vi "I(V)_K2636B_PK.vi"() -> ()   [LabVIEW 2016]
uses:
  <instrlib>/Keithley 2600 Series/Public/Configure/Source/Configure Source (Limit).vi
  <instrlib>/Keithley 2600 Series/Public/Configure/Source/Configure Source (Range).vi
  <instrlib>/Keithley 2600 Series/Public/Data/Read Measurement (Current and Voltage).vi
  <instrlib>/Keithley 2600 Series/Keithley 2600 Series.lvlib
panel:
  in  "4-point sense":bool
  out "Resistance (ohm)":dbl=129228.0822461563 format="%#_13g"
  out "R vs V":cluster{dbl, "Field Reading":dbl}[](graph)=[{9.24826e-05, "Field Reading"=321246.1833983473}, {0.00208223, "Field Reading"=133422.3999282341}, {0.00408287, "Field Reading"=132230.99543994194}, {0.00608664, "Field Reading"=131799.94326658855}, {0.00808966, "Field Reading"=131627.15245472992}, {0.0100896, "Field Reading"=131526.7352701163}, {0.0120913, "Field Reading"=131453.46460596466}, {0.0140768, "Field Reading"=131503.57326358074}, {0.0160766, "Field Reading"=131110.1868389075}, {0.0180795, "Field Reading"=131062.15475620893}, {0.0200782, "Field Reading"=131023.68165177728}, {0.0220798, "Field Reading"=130975.9815872677}, {0.0240771, "Field Reading"=130942.0479018469}, {0.0260761, "Field Reading"=130887.03281700182}, {0.0280696, "Field Reading"=130884.40322482875}, {0.0300689, "Field Reading"=130827.06439781236}, {0.0320729, "Field Reading"=130811.55377186114}, {0.0340708, "Field Reading"=130758.89807416276}, {0.0360752, "Field Reading"=130716.71860279731}, {0.0380763, "Field Reading"=130666.78105696639}, {0.0400745, "Field Reading"=130596.66228894892}, {0.042069, "Field Reading"=130525.02900969888}, {0.0440687, "Field Reading"=130462.21161731142}, {0.0460705, "Field Reading"=130389.80666744027}, {0.0480758, "Field Reading"=130307.55595068047}, {0.0500756, "Field Reading"=130219.03580558003}, {0.0520796, "Field Reading"=130135.55891502892}, {0.0540786, "Field Reading"=130028.82925339688}, {0.0560762, "Field Reading"=129906.75639674284}, {0.0580758, "Field Reading"=129809.94253348859}, {0.0600795, "Field Reading"=129706.1509465735}, {0.06208, "Field Reading"=129574.12524942185}, {0.0640783, "Field Reading"=129469.68150987315}, {0.0660839, "Field Reading"=129344.46893214904}, {0.0680779, "Field Reading"=129205.08333681281}, {0.0700804, "Field Reading"=129056.75665721338}, {0.0720784, "Field Reading"=128949.2939654756}, {0.0740798, "Field Reading"=128777.32483854984}, {0.0760786, "Field Reading"=128620.215114844}, {0.0780784, "Field Reading"=128483.7195219281}, {0.080081, "Field Reading"=128312.52233183626}, {0.082076, "Field Reading"=128154.84257796154}, {0.0840742, "Field Reading"=127980.8441716596}, {0.0860755, "Field Reading"=127813.893954063}, {0.0880753, "Field Reading"=127647.5822767932}, {0.0900754, "Field Reading"=127475.23036012742}, {0.0920787, "Field Reading"=127295.51279747175}, {0.094079, "Field Reading"=127096.34188847069}, {0.0960754, "Field Reading"=126929.56577916528}, {0.0980756, "Field Reading"=126726.5785002229}, {0.100075, "Field Reading"=126544.74366707256}, {0.102075, "Field Reading"=126340.60908365152}, {0.104078, "Field Reading"=126112.5025597404}, {0.106077, "Field Reading"=125926.55026520349}, {0.108078, "Field Reading"=125701.17969157979}, {0.110074, "Field Reading"=125495.65962919302}, {0.112071, "Field Reading"=125291.5094993527}, {0.114072, "Field Reading"=125059.33828358054}, {0.116073, "Field Reading"=124826.99213116657}, {0.118074, "Field Reading"=124620.17307126023}, {0.120074, "Field Reading"=124379.39267753281}, {0.122073, "Field Reading"=124152.80783688347}, {0.124068, "Field Reading"=123908.15847556652}, {0.12607, "Field Reading"=123681.70625226868}, {0.12807, "Field Reading"=123435.01517999133}, {0.130073, "Field Reading"=123193.85512956508}, {0.13207, "Field Reading"=122948.45418408289}, {0.134072, "Field Reading"=122693.4128887018}, {0.136065, "Field Reading"=122423.3644943901}, {0.138062, "Field Reading"=122188.49288881414}, {0.140062, "Field Reading"=121878.88860849815}, {0.142063, "Field Reading"=121633.44635090242}, {0.144064, "Field Reading"=121365.08765574585}, {0.146064, "Field Reading"=121085.31116066618}, {0.148066, "Field Reading"=120833.70737001886}, {0.150064, "Field Reading"=120578.85306099491}, {0.152064, "Field Reading"=120319.0277250285}, {0.154064, "Field Reading"=120031.47569593231}, {0.156068, "Field Reading"=119745.5747968665}, {0.158069, "Field Reading"=119474.99300847296}, {0.160068, "Field Reading"=119184.23266792252}, {0.162069, "Field Reading"=118894.74958367874}, {0.164067, "Field Reading"=118602.07902612517}, {0.166065, "Field Reading"=118316.99392972156}, {0.168064, "Field Reading"=118033.24741725015}, {0.170065, "Field Reading"=117718.11058504305}, {0.172066, "Field Reading"=117415.92968664701}, {0.174067, "Field Reading"=117115.8866431628}, {0.176067, "Field Reading"=116815.72696752963}, {0.178062, "Field Reading"=116516.70909102805}, {0.180063, "Field Reading"=116204.1638163584}, {0.182065, "Field Reading"=115904.4320800601}, {0.184064, "Field Reading"=115589.77386193082}, {0.186063, "Field Reading"=115279.24065377133}, {0.188066, "Field Reading"=114950.55193574808}, {0.190068, "Field Reading"=114624.46778998661}, {0.192063, "Field Reading"=114307.56503573916}, {0.194061, "Field Reading"=113989.25078563248}, {0.196063, "Field Reading"=113656.41575606503}, {0.198066, "Field Reading"=113329.51879613205}, {0.200067, "Field Reading"=113007.3034755054}, {0.202094, "Field Reading"=112660.62001415963}, {0.2041, "Field Reading"=112315.65045124368}, {0.206103, "Field Reading"=111972.94434031457}, {0.20811, "Field Reading"=111652.38664956999}, {0.210077, "Field Reading"=111303.20064850089}, {0.212084, "Field Reading"=110989.93112976493}, {0.214085, "Field Reading"=110626.80859859445}, {0.216093, "Field Reading"=110267.2830812565}, {0.218084, "Field Reading"=109914.72289982461}, {0.220093, "Field Reading"=109567.14374611077}, {0.222097, "Field Reading"=109202.43287229385}, {0.224105, "Field Reading"=108854.35893450427}, {0.226104, "Field Reading"=108514.98833760475}, {0.228108, "Field Reading"=108141.37056439188}, {0.23008, "Field Reading"=107803.17299672955}, {0.232083, "Field Reading"=107437.37761379892}, {0.234082, "Field Reading"=107060.3032312653}, {0.236089, "Field Reading"=106702.06996293954}, {0.238094, "Field Reading"=106322.34209774222}, {0.240097, "Field Reading"=105957.24587154345}, {0.242102, "Field Reading"=105580.77669479515}, {0.244106, "Field Reading"=105224.45319976204}, {0.246111, "Field Reading"=104835.1507922985}, {0.248119, "Field Reading"=104436.41904377071}, {0.250125, "Field Reading"=104089.93870085767}, {0.252088, "Field Reading"=103727.53868879845}, {0.254094, "Field Reading"=103335.19050969325}, {0.256097, "Field Reading"=102949.01531992556}, {0.258105, "Field Reading"=102551.62247748158}, {0.260109, "Field Reading"=102170.60840668858}, {0.262107, "Field Reading"=101770.94577279399}, {0.264109, "Field Reading"=101381.1316988534}, {0.266118, "Field Reading"=100992.39856851725}, {0.268115, "Field Reading"=100595.43462600552}, {0.27012, "Field Reading"=100202.54178815465}, {0.272085, "Field Reading"=99831.95312299344}, {0.274093, "Field Reading"=99428.66056270585}, {0.276096, "Field Reading"=99019.82935777842}, {0.2781, "Field Reading"=98626.8140099017}, {0.280098, "Field Reading"=98219.3452464443}, {0.282103, "Field Reading"=97817.59172252139}, {0.284104, "Field Reading"=97427.35060321119}, {0.28611, "Field Reading"=96994.00292226172}, {0.288119, "Field Reading"=96597.67926052833}, {0.29012, "Field Reading"=96211.81722009796}, {0.292129, "Field Reading"=95793.50531386393}, {0.294094, "Field Reading"=95378.22893187826}, {0.296091, "Field Reading"=94976.15099132966}, {0.298098, "Field Reading"=94562.53826461827}, {0.300094, "Field Reading"=94141.52568160644}, {0.302104, "Field Reading"=93737.56930934229}, {0.304106, "Field Reading"=93326.13172197278}, {0.306113, "Field Reading"=92900.58451135943}, {0.308113, "Field Reading"=92468.39070973474}, {0.310119, "Field Reading"=92046.93185798156}, {0.312124, "Field Reading"=91641.61225160897}, {0.314088, "Field Reading"=91218.20600245116}, {0.316094, "Field Reading"=90804.47222669086}, {0.318097, "Field Reading"=90406.22077970063}, {0.320102, "Field Reading"=89978.46826739826}, {0.322106, "Field Reading"=89544.52957333007}, {0.324107, "Field Reading"=89123.63196392234}, {0.326113, "Field Reading"=88690.44705165652}, {0.328116, "Field Reading"=88285.34066631868}, {0.33012, "Field Reading"=87849.97485210645}, {0.332121, "Field Reading"=87440.07140092726}, {0.334123, "Field Reading"=87014.82353431392}, {0.33609, "Field Reading"=86605.06297800409}, {0.338095, "Field Reading"=86185.18490194727}, {0.340103, "Field Reading"=85757.69190036965}, {0.342109, "Field Reading"=85336.73573746611}, {0.34411, "Field Reading"=84911.13090640801}, {0.346114, "Field Reading"=84463.1644707783}, {0.348119, "Field Reading"=84029.07184443522}, {0.350126, "Field Reading"=83601.39826744731}, {0.352124, "Field Reading"=83178.96313304183}, {0.354127, "Field Reading"=82744.78649453823}, {0.356091, "Field Reading"=82317.38186660132}, {0.358103, "Field Reading"=81892.17125634025}, {0.360106, "Field Reading"=81455.7282712944}, {0.362108, "Field Reading"=81034.78757091226}, {0.364112, "Field Reading"=80599.43996192627}, {0.366113, "Field Reading"=80163.29873070162}, {0.368121, "Field Reading"=79741.83402254131}, {0.370123, "Field Reading"=79323.91335563666}, {0.372125, "Field Reading"=78905.23949873837}, {0.374122, "Field Reading"=78477.3643560452}, {0.376098, "Field Reading"=78042.55531069858}, {0.378101, "Field Reading"=77644.22978195603}, {0.380109, "Field Reading"=77197.36141969917}, {0.382109, "Field Reading"=76788.07913748581}, {0.384122, "Field Reading"=76341.00873270452}, {0.386122, "Field Reading"=75917.70447065115}, {0.388125, "Field Reading"=75482.06419743483}, {0.39013, "Field Reading"=75072.35333056234}, {0.392133, "Field Reading"=74630.30561402574}, {0.394136, "Field Reading"=74217.1288258533}, {0.39614, "Field Reading"=73795.3350260521}, {0.398104, "Field Reading"=73389.04281814043}, {0.400107, "Field Reading"=72968.81782005595}, {0.40211, "Field Reading"=72549.37691359785}, {0.40412, "Field Reading"=72130.79641594974}, {0.40612, "Field Reading"=71711.09321806444}, {0.408124, "Field Reading"=71287.91041413028}, {0.410125, "Field Reading"=70871.400700549}, {0.412135, "Field Reading"=70465.72503774324}, {0.414137, "Field Reading"=70025.71832934003}, {0.416143, "Field Reading"=69611.94639045573}, {0.418111, "Field Reading"=69209.6960547704}, {0.420117, "Field Reading"=68799.2309733035}, {0.422119, "Field Reading"=68364.2235236195}, {0.42412, "Field Reading"=67960.32496354575}, {0.426121, "Field Reading"=67564.2550222772}, {0.428125, "Field Reading"=67151.279972018}, {0.430128, "Field Reading"=66733.58725922937}, {0.432133, "Field Reading"=66333.61680180028}, {0.434134, "Field Reading"=65937.3272337349}, {0.436139, "Field Reading"=65541.44626112047}, {0.438137, "Field Reading"=65136.632656550355}, {0.440108, "Field Reading"=64742.996600355706}, {0.44211, "Field Reading"=64342.660212656345}, {0.44411, "Field Reading"=63933.376040999356}, {0.446114, "Field Reading"=63529.36485445382}, {0.448117, "Field Reading"=63144.686169710585}, {0.450123, "Field Reading"=62747.85600374712}, {0.452128, "Field Reading"=62336.68826692403}, {0.45413, "Field Reading"=61937.23489859658}, {0.456133, "Field Reading"=61550.927987520685}, {0.458137, "Field Reading"=61165.427035311805}, {0.460102, "Field Reading"=60772.11020031859}, {0.4621, "Field Reading"=60378.55169872657}, {0.464111, "Field Reading"=59998.862362691696}, {0.466115, "Field Reading"=59625.094180568296}, {0.468126, "Field Reading"=59241.00804094122}, {0.470129, "Field Reading"=58849.10223415015}, {0.472136, "Field Reading"=58461.759439721245}, {0.474135, "Field Reading"=58103.64012470343}, {0.476139, "Field Reading"=57723.19382784597}, {0.478142, "Field Reading"=57346.646277472944}, {0.480145, "Field Reading"=56982.72639342997}, {0.482113, "Field Reading"=56622.85100875452}, {0.484118, "Field Reading"=56250.14523872599}, {0.486126, "Field Reading"=55881.626032708715}, {0.488123, "Field Reading"=55509.90283666005}, {0.490129, "Field Reading"=55163.2740803101}, {0.49213, "Field Reading"=54799.41696351123}, {0.494141, "Field Reading"=54432.26493678737}, {0.49614, "Field Reading"=54083.22105511007}, {0.498144, "Field Reading"=53717.05120407872}, {0.500151, "Field Reading"=53362.07613962987}, {0.498148, "Field Reading"=53694.09066215971}, {0.496145, "Field Reading"=54062.78603495619}, {0.494146, "Field Reading"=54420.82622529071}, {0.492136, "Field Reading"=54795.02082080745}, {0.490135, "Field Reading"=55146.50866855613}, {0.488125, "Field Reading"=55511.077196362225}, {0.486143, "Field Reading"=55867.39648322805}, {0.484113, "Field Reading"=56244.9243252475}, {0.48212, "Field Reading"=56602.99827298162}, {0.480148, "Field Reading"=56968.816813909405}, {0.478147, "Field Reading"=57345.664057721406}, {0.476143, "Field Reading"=57702.83240664886}, {0.47414, "Field Reading"=58066.46769873627}, {0.472135, "Field Reading"=58421.05328283172}, {0.470131, "Field Reading"=58798.05245075785}, {0.46813, "Field Reading"=59195.967699104964}, {0.466119, "Field Reading"=59575.23223296405}, {0.464119, "Field Reading"=59952.92835007667}, {0.462114, "Field Reading"=60343.48124720883}, {0.460119, "Field Reading"=60748.11762546853}, {0.458148, "Field Reading"=61120.3829329107}, {0.456138, "Field Reading"=61521.301375313415}, {0.454138, "Field Reading"=61888.60982367106}, {0.452139, "Field Reading"=62289.25289652417}, {0.450134, "Field Reading"=62664.91628371239}, {0.448129, "Field Reading"=63052.73095912461}, {0.446123, "Field Reading"=63421.634746610864}, {0.444124, "Field Reading"=63816.42095582953}, {0.442118, "Field Reading"=64218.96016291575}, {0.440114, "Field Reading"=64609.20090312011}, {0.438145, "Field Reading"=65016.515852547425}, {0.436145, "Field Reading"=65423.28744725501}, {0.43414, "Field Reading"=65803.81326837934}, {0.432137, "Field Reading"=66215.71511752627}, {0.430135, "Field Reading"=66612.72213403539}, {0.428127, "Field Reading"=67016.41571663597}, {0.426126, "Field Reading"=67419.77283406825}, {0.424124, "Field Reading"=67825.98127014995}, {0.422123, "Field Reading"=68233.58829957132}, {0.420119, "Field Reading"=68652.27991737914}, {0.418111, "Field Reading"=69060.1721090795}, {0.416145, "Field Reading"=69472.36097013729}, {0.414139, "Field Reading"=69883.78548491337}, {0.41214, "Field Reading"=70283.56264367425}, {0.410131, "Field Reading"=70709.43738437959}, {0.408128, "Field Reading"=71132.67660817491}, {0.406125, "Field Reading"=71517.50054590152}, {0.404124, "Field Reading"=71928.91901224197}, {0.40212, "Field Reading"=72353.41111103114}, {0.400116, "Field Reading"=72769.00357192222}, {0.398111, "Field Reading"=73192.93278423297}, {0.396139, "Field Reading"=73603.46483787836}, {0.394134, "Field Reading"=74025.08860269742}, {0.392128, "Field Reading"=74427.22084192984}, {0.390125, "Field Reading"=74849.72496743161}, {0.388125, "Field Reading"=75278.85907797581}, {0.38612, "Field Reading"=75678.49379962409}, {0.384116, "Field Reading"=76096.32787612724}, {0.382109, "Field Reading"=76527.56108942558}, {0.380107, "Field Reading"=76957.19954648525}, {0.378106, "Field Reading"=77366.27366887515}, {0.376101, "Field Reading"=77782.51149362292}, {0.37413, "Field Reading"=78219.31011124607}, {0.372128, "Field Reading"=78653.21003963012}, {0.370126, "Field Reading"=79068.50555854631}, {0.368119, "Field Reading"=79481.59343625176}, {0.366114, "Field Reading"=79899.00070053534}, {0.364111, "Field Reading"=80318.48482575762}, {0.36211, "Field Reading"=80756.92191036922}, {0.360107, "Field Reading"=81184.17018360207}, {0.358103, "Field Reading"=81609.4311544413}, {0.356093, "Field Reading"=82039.62677110931}, {0.354124, "Field Reading"=82471.79706931725}, {0.352115, "Field Reading"=82891.15614230023}, {0.350114, "Field Reading"=83289.67996250805}, {0.34811, "Field Reading"=83734.63546051523}, {0.346107, "Field Reading"=84145.22963816582}, {0.344101, "Field Reading"=84579.15784868215}, {0.3421, "Field Reading"=85005.19324331712}, {0.340095, "Field Reading"=85423.74669389415}, {0.338091, "Field Reading"=85859.58371849699}, {0.336087, "Field Reading"=86269.05898660095}, {0.334123, "Field Reading"=86675.55585532068}, {0.332117, "Field Reading"=87107.85766554497}, {0.330117, "Field Reading"=87542.36344253687}, {0.328107, "Field Reading"=87955.85412667945}, {0.326111, "Field Reading"=88396.3688506149}, {0.324107, "Field Reading"=88779.6553528237}, {0.322109, "Field Reading"=89197.96077171664}, {0.320099, "Field Reading"=89606.10700698993}, {0.318093, "Field Reading"=90027.93446297622}, {0.316093, "Field Reading"=90433.20783218705}, {0.314091, "Field Reading"=90802.41452880263}, {0.31212, "Field Reading"=91223.41436041023}, {0.310117, "Field Reading"=91681.15273638899}, {0.308112, "Field Reading"=92070.7491774915}, {0.306114, "Field Reading"=92490.79213335468}, {0.304108, "Field Reading"=92900.23797231702}, {0.302107, "Field Reading"=93307.41006127694}, {0.300098, "Field Reading"=93718.53646958889}, {0.298095, "Field Reading"=94131.5969799071}, {0.296094, "Field Reading"=94545.55904667026}, {0.294092, "Field Reading"=94961.20401553776}, {0.29212, "Field Reading"=95340.98141288206}, {0.290125, "Field Reading"=95759.0420300092}, {0.28812, "Field Reading"=96165.01451887454}, {0.286114, "Field Reading"=96573.67559448467}, {0.284114, "Field Reading"=96982.4614103238}, {0.282104, "Field Reading"=97383.35565650847}, {0.280102, "Field Reading"=97775.37306920325}, {0.2781, "Field Reading"=98178.69864682147}, {0.276096, "Field Reading"=98568.39910605272}, {0.274095, "Field Reading"=98959.48039006848}, {0.272086, "Field Reading"=99349.68433582723}, {0.270118, "Field Reading"=99741.52382781057}, {0.268115, "Field Reading"=100140.80929864271}, {0.266113, "Field Reading"=100537.23020427593}, {0.264107, "Field Reading"=100920.91235283551}, {0.262103, "Field Reading"=101298.58585546275}, {0.260103, "Field Reading"=101689.32919439209}, {0.258096, "Field Reading"=102078.78500237304}, {0.256092, "Field Reading"=102463.03053581716}, {0.254086, "Field Reading"=102848.42278252491}, {0.252086, "Field Reading"=103221.28908889153}, {0.250122, "Field Reading"=103595.92445328031}, {0.248116, "Field Reading"=103962.55745645461}, {0.24611, "Field Reading"=104336.50866326665}, {0.244101, "Field Reading"=104720.7814772391}, {0.242097, "Field Reading"=105074.08661232781}, {0.240094, "Field Reading"=105459.33718402038}, {0.238089, "Field Reading"=105822.97722545202}, {0.236082, "Field Reading"=106195.43068431776}, {0.23408, "Field Reading"=106538.98494854651}, {0.232076, "Field Reading"=106889.34127985704}, {0.230075, "Field Reading"=107247.57256662332}, {0.228099, "Field Reading"=107611.12631271053}, {0.226096, "Field Reading"=107967.58527489005}, {0.224093, "Field Reading"=108331.8024925311}, {0.222093, "Field Reading"=108661.91429088649}, {0.220095, "Field Reading"=109021.0666574204}, {0.21809, "Field Reading"=109352.27990653735}, {0.216086, "Field Reading"=109721.185532723}, {0.214077, "Field Reading"=110053.97902529303}, {0.212077, "Field Reading"=110394.09918327616}, {0.210073, "Field Reading"=110734.91892803677}, {0.208101, "Field Reading"=111061.83355214704}, {0.206095, "Field Reading"=111409.92929271088}, {0.204095, "Field Reading"=111727.57729701322}, {0.202089, "Field Reading"=112072.42679680568}, {0.200064, "Field Reading"=112420.13699630818}, {0.198062, "Field Reading"=112749.19449409675}, {0.196061, "Field Reading"=113064.71517709884}, {0.194063, "Field Reading"=113401.5859380935}, {0.192065, "Field Reading"=113732.72380591447}, {0.190067, "Field Reading"=114031.0775137989}, {0.188066, "Field Reading"=114351.55627709576}, {0.186066, "Field Reading"=114665.86141445018}, {0.184067, "Field Reading"=114983.66451983684}, {0.182063, "Field Reading"=115313.67767679007}, {0.180062, "Field Reading"=115599.98202397232}, {0.178062, "Field Reading"=115906.16171741762}, {0.176065, "Field Reading"=116219.12418973689}, {0.174063, "Field Reading"=116519.73089667637}, {0.17206, "Field Reading"=116821.1291034389}, {0.17006, "Field Reading"=117123.63203096481}, {0.16806, "Field Reading"=117435.78276546384}, {0.166061, "Field Reading"=117698.63207881495}, {0.164059, "Field Reading"=117983.07120306646}, {0.162066, "Field Reading"=118292.03313747673}, {0.160064, "Field Reading"=118575.58764047442}, {0.158063, "Field Reading"=118866.7042677195}, {0.156057, "Field Reading"=119133.84684677808}, {0.154056, "Field Reading"=119425.10736600567}, {0.152056, "Field Reading"=119689.55148690983}, {0.150057, "Field Reading"=119994.72223777119}, {0.148063, "Field Reading"=120266.91143024237}, {0.146063, "Field Reading"=120523.970624639}, {0.144062, "Field Reading"=120800.63057623935}, {0.142062, "Field Reading"=121053.21460525756}, {0.140061, "Field Reading"=121324.80964631894}, {0.138061, "Field Reading"=121590.36866115936}, {0.136064, "Field Reading"=121849.08566618308}, {0.134067, "Field Reading"=122099.98087449113}, {0.132062, "Field Reading"=122348.73400717074}, {0.130064, "Field Reading"=122613.97488593085}, {0.128063, "Field Reading"=122850.45518643939}, {0.126063, "Field Reading"=123081.95504872}, {0.124066, "Field Reading"=123318.68874619804}, {0.122069, "Field Reading"=123552.24469759462}, {0.120073, "Field Reading"=123783.91808012404}, {0.118072, "Field Reading"=124004.23877894599}, {0.116074, "Field Reading"=124244.83749288188}, {0.114072, "Field Reading"=124487.22355906956}, {0.112071, "Field Reading"=124715.2562554598}, {0.110071, "Field Reading"=124913.89338099697}, {0.108072, "Field Reading"=125139.38534968787}, {0.106072, "Field Reading"=125349.94392624972}, {0.104071, "Field Reading"=125555.71775509934}, {0.10207, "Field Reading"=125773.53124561018}, {0.100074, "Field Reading"=125973.21020585166}, {0.0980714, "Field Reading"=126166.54466581845}, {0.0960723, "Field Reading"=126345.7532430641}, {0.0940741, "Field Reading"=126549.99159239951}, {0.0920758, "Field Reading"=126745.863502464}, {0.0900749, "Field Reading"=126912.88898156784}, {0.0880718, "Field Reading"=127101.49006025183}, {0.0860697, "Field Reading"=127278.54830671767}, {0.0840724, "Field Reading"=127474.16701413896}, {0.0820718, "Field Reading"=127624.5894705414}, {0.0800771, "Field Reading"=127776.21757210011}, {0.078074, "Field Reading"=127924.31436932465}, {0.0760751, "Field Reading"=128086.35947307455}, {0.0740699, "Field Reading"=128246.90896309802}, {0.0720729, "Field Reading"=128393.92028389109}, {0.0700725, "Field Reading"=128523.40007189864}, {0.0680684, "Field Reading"=128663.75195873287}, {0.066073, "Field Reading"=128794.25822397918}, {0.0640697, "Field Reading"=128920.91860860537}, {0.0620658, "Field Reading"=129058.53877632496}, {0.0600666, "Field Reading"=129172.42817911835}, {0.0580685, "Field Reading"=129297.4073051471}, {0.0560677, "Field Reading"=129403.52383458194}, {0.054073, "Field Reading"=129523.6133334611}, {0.0520688, "Field Reading"=129616.59289942594}, {0.0500681, "Field Reading"=129722.53817075728}, {0.0480689, "Field Reading"=129802.98226948439}, {0.0460666, "Field Reading"=129881.78109343324}, {0.0440633, "Field Reading"=129963.75091065146}, {0.042061, "Field Reading"=130028.19374544016}, {0.0400637, "Field Reading"=130096.80048578842}, {0.0380634, "Field Reading"=130188.69860553884}, {0.0360641, "Field Reading"=130237.1520091293}, {0.0340635, "Field Reading"=130279.88556742035}, {0.0320607, "Field Reading"=130328.5785714576}, {0.0300555, "Field Reading"=130360.3881035926}, {0.0280551, "Field Reading"=130403.31689450174}, {0.026058, "Field Reading"=130400.18815899435}, {0.0240593, "Field Reading"=130440.8878479338}, {0.0220574, "Field Reading"=130481.64404954866}, {0.0200566, "Field Reading"=130487.62239354607}, {0.01806, "Field Reading"=130508.30310300473}, {0.0160547, "Field Reading"=130503.73513465183}, {0.0140561, "Field Reading"=130540.69616256176}, {0.012063, "Field Reading"=130847.06198829395}, {0.0100592, "Field Reading"=130791.15438224221}, {0.00805471, "Field Reading"=130763.58618450422}, {0.00605381, "Field Reading"=130647.99468241225}, {0.00404904, "Field Reading"=130641.58613902917}, {0.00205326, "Field Reading"=130915.97699537102}, {4.89712e-05, "Field Reading"=171453.9795464651}, {-0.00196376, "Field Reading"=126201.60020564894}, {-0.0039638, "Field Reading"=128450.83202359156}, {-0.00596104, "Field Reading"=129070.14258030291}, {-0.0079607, "Field Reading"=129374.32860465153}, {-0.00995808, "Field Reading"=129545.26827935656}, {-0.0119533, "Field Reading"=129604.85228041567}, {-0.0139638, "Field Reading"=129746.1532743626}, {-0.0159607, "Field Reading"=129333.83033377363}, {-0.0179633, "Field Reading"=129288.18194904276}, {-0.0199615, "Field Reading"=129234.10591738962}, {-0.0219611, "Field Reading"=129181.42139504243}, {-0.0239586, "Field Reading"=129067.11774561087}, {-0.0259606, "Field Reading"=128979.4661088947}, {-0.0279626, "Field Reading"=128884.25923792053}, {-0.0299578, "Field Reading"=128750.52109970304}, {-0.031959, "Field Reading"=128635.08112394193}, {-0.0339592, "Field Reading"=128506.28734470847}, {-0.0359603, "Field Reading"=128360.41991640223}, {-0.0379647, "Field Reading"=128220.13576952953}, {-0.0399635, "Field Reading"=128073.3633298722}, {-0.0419601, "Field Reading"=127915.43456391184}, {-0.0439643, "Field Reading"=127758.25944943783}, {-0.0459585, "Field Reading"=127558.68140652192}, {-0.0479606, "Field Reading"=127366.44748722634}, {-0.0499626, "Field Reading"=127197.64762789752}, {-0.0519609, "Field Reading"=127010.22712828885}, {-0.0539638, "Field Reading"=126805.3688751868}, {-0.0559645, "Field Reading"=126618.52110780036}, {-0.0579646, "Field Reading"=126406.80745645025}, {-0.0599606, "Field Reading"=126198.03801477909}, {-0.0619605, "Field Reading"=125995.64427869295}, {-0.0639597, "Field Reading"=125769.4962314201}, {-0.0659617, "Field Reading"=125549.98077589259}, {-0.06796, "Field Reading"=125342.82072988771}, {-0.0699609, "Field Reading"=125117.4078352964}, {-0.0719576, "Field Reading"=124879.77577813837}, {-0.0739591, "Field Reading"=124642.04579926253}, {-0.0759554, "Field Reading"=124410.3825736295}, {-0.0779573, "Field Reading"=124182.69315012194}, {-0.0799575, "Field Reading"=123916.70231165497}, {-0.0819596, "Field Reading"=123683.29316675142}, {-0.0839633, "Field Reading"=123435.14323265052}, {-0.0859642, "Field Reading"=123167.23189583163}, {-0.0879685, "Field Reading"=122911.33103350953}, {-0.0899625, "Field Reading"=122676.52669803948}, {-0.091961, "Field Reading"=122403.80571069571}, {-0.0939611, "Field Reading"=122170.99318029633}, {-0.0959609, "Field Reading"=121860.99138752093}, {-0.097957, "Field Reading"=121585.42518965722}, {-0.0999584, "Field Reading"=121320.36930725155}, {-0.101958, "Field Reading"=121045.26464627756}, {-0.10396, "Field Reading"=120857.86296885317}, {-0.105956, "Field Reading"=120578.83668211324}, {-0.107955, "Field Reading"=120206.84195230475}, {-0.109957, "Field Reading"=119920.34175394283}, {-0.111957, "Field Reading"=119639.27727220269}, {-0.113957, "Field Reading"=119327.45127194516}, {-0.115961, "Field Reading"=119060.1353224432}, {-0.117958, "Field Reading"=118754.24722766147}, {-0.119958, "Field Reading"=118475.86690501824}, {-0.121958, "Field Reading"=118179.79204821844}, {-0.123962, "Field Reading"=117869.33411936979}, {-0.12596, "Field Reading"=117564.7044548772}, {-0.127961, "Field Reading"=117277.05984785994}, {-0.129961, "Field Reading"=116968.17510890306}, {-0.131962, "Field Reading"=116644.27394547961}, {-0.133958, "Field Reading"=116356.71910151398}, {-0.135959, "Field Reading"=116055.48442168161}, {-0.137961, "Field Reading"=115736.1811363808}, {-0.139958, "Field Reading"=115424.51857655354}, {-0.141961, "Field Reading"=115094.49259382374}, {-0.143963, "Field Reading"=114776.48709628556}, {-0.145961, "Field Reading"=114463.95382576442}, {-0.147961, "Field Reading"=114142.77779492085}, {-0.14996, "Field Reading"=113821.63187855788}, {-0.151959, "Field Reading"=113496.2543599549}, {-0.15396, "Field Reading"=113174.26013319808}, {-0.155959, "Field Reading"=112840.4190663618}, {-0.15796, "Field Reading"=112527.15939447908}, {-0.15996, "Field Reading"=112200.66495517865}, {-0.161958, "Field Reading"=111870.30730868324}, {-0.163955, "Field Reading"=111549.19036603619}, {-0.165959, "Field Reading"=111193.07484606674}, {-0.167959, "Field Reading"=110869.14906959397}, {-0.16996, "Field Reading"=110544.52740848661}, {-0.171962, "Field Reading"=110186.84642198074}, {-0.173959, "Field Reading"=109844.09827680924}, {-0.17596, "Field Reading"=109512.31048818742}, {-0.177961, "Field Reading"=109169.15111585509}, {-0.179957, "Field Reading"=108798.4571110735}, {-0.181956, "Field Reading"=108469.84762858575}, {-0.183955, "Field Reading"=108159.197544656}, {-0.185953, "Field Reading"=107778.84682261842}, {-0.187954, "Field Reading"=107436.66544722884}, {-0.189952, "Field Reading"=107103.30750927524}, {-0.191953, "Field Reading"=106795.40889845832}, {-0.193951, "Field Reading"=106403.95439932411}, {-0.195952, "Field Reading"=106039.22247716351}, {-0.197953, "Field Reading"=105694.43851181069}, {-0.199955, "Field Reading"=105351.4789407686}, {-0.20198, "Field Reading"=104986.30364837541}, {-0.203947, "Field Reading"=104628.9836038661}, {-0.205948, "Field Reading"=104264.7982017375}, {-0.207951, "Field Reading"=103892.38609112709}, {-0.209952, "Field Reading"=103566.97135471905}, {-0.211962, "Field Reading"=103175.65396859394}, {-0.213962, "Field Reading"=102832.2335379129}, {-0.215967, "Field Reading"=102445.30671878261}, {-0.217971, "Field Reading"=102101.79685597046}, {-0.219975, "Field Reading"=101735.71606959515}, {-0.221975, "Field Reading"=101393.63432058615}, {-0.223982, "Field Reading"=100987.86695582779}, {-0.22595, "Field Reading"=100631.535816721}, {-0.22795, "Field Reading"=100231.72678225157}, {-0.229955, "Field Reading"=99885.76045313572}, {-0.231961, "Field Reading"=99510.9416090021}, {-0.233959, "Field Reading"=99121.30930844415}, {-0.235963, "Field Reading"=98771.85565327317}, {-0.237971, "Field Reading"=98409.13414220612}, {-0.239972, "Field Reading"=98004.15749472145}, {-0.241978, "Field Reading"=97645.7960066502}, {-0.24398, "Field Reading"=97261.31154076141}, {-0.245986, "Field Reading"=96883.40639388104}, {-0.247953, "Field Reading"=96510.93543829331}, {-0.249964, "Field Reading"=96120.03660778145}, {-0.251966, "Field Reading"=95731.76291793314}, {-0.253968, "Field Reading"=95374.50475993767}, {-0.255967, "Field Reading"=94976.36416257895}, {-0.257976, "Field Reading"=94591.98826656888}, {-0.259975, "Field Reading"=94220.46810330456}, {-0.261979, "Field Reading"=93830.00365321663}, {-0.26398, "Field Reading"=93464.0985696077}, {-0.265988, "Field Reading"=93058.11146485675}, {-0.267989, "Field Reading"=92657.29913631555}, {-0.269958, "Field Reading"=92284.49926160913}, {-0.27196, "Field Reading"=91907.87583852925}, {-0.273967, "Field Reading"=91509.92868714198}, {-0.27597, "Field Reading"=91098.75055705018}, {-0.277973, "Field Reading"=90721.9623956841}, {-0.279978, "Field Reading"=90337.04819860225}, {-0.28198, "Field Reading"=89945.19971164459}, {-0.283984, "Field Reading"=89556.04190449762}, {-0.285989, "Field Reading"=89161.47577271055}, {-0.287992, "Field Reading"=88774.62947892777}, {-0.289996, "Field Reading"=88395.8971545273}, {-0.291996, "Field Reading"=87976.83646629566}, {-0.293969, "Field Reading"=87591.92162377984}, {-0.29597, "Field Reading"=87196.18183425155}, {-0.297976, "Field Reading"=86803.11584197066}, {-0.299977, "Field Reading"=86400.1497717421}, {-0.301984, "Field Reading"=86009.84323733138}, {-0.303985, "Field Reading"=85610.76721171124}, {-0.305994, "Field Reading"=85219.66774817929}, {-0.307994, "Field Reading"=84814.82195424866}, {-0.309994, "Field Reading"=84436.66038373118}, {-0.312002, "Field Reading"=84021.47919943124}, {-0.314005, "Field Reading"=83624.05991009226}, {-0.31597, "Field Reading"=83244.63600725034}, {-0.317976, "Field Reading"=82824.3678304629}, {-0.319977, "Field Reading"=82417.5314690178}, {-0.321985, "Field Reading"=82029.7970559612}, {-0.323984, "Field Reading"=81639.93498721163}, {-0.325988, "Field Reading"=81221.65857742254}, {-0.327989, "Field Reading"=80837.63413828629}, {-0.329999, "Field Reading"=80442.43473173586}, {-0.332, "Field Reading"=80019.86035088227}, {-0.33401, "Field Reading"=79625.72262947731}, {-0.336008, "Field Reading"=79234.64924174716}, {-0.337976, "Field Reading"=78834.10540261898}, {-0.339982, "Field Reading"=78439.52453902805}, {-0.341988, "Field Reading"=78015.50783718369}, {-0.343988, "Field Reading"=77634.76533847908}, {-0.345992, "Field Reading"=77237.77058958785}, {-0.348, "Field Reading"=76845.61979967142}, {-0.350002, "Field Reading"=76440.17934947595}, {-0.352004, "Field Reading"=76020.54259045693}, {-0.354007, "Field Reading"=75640.58186542225}, {-0.356012, "Field Reading"=75242.46913788986}, {-0.358017, "Field Reading"=74832.41887443172}, {-0.359986, "Field Reading"=74449.87673929946}, {-0.361982, "Field Reading"=74055.99484446445}, {-0.363986, "Field Reading"=73656.02930165733}, {-0.365991, "Field Reading"=73247.12908222694}, {-0.367996, "Field Reading"=72859.09728973091}, {-0.369992, "Field Reading"=72464.04628398294}, {-0.371998, "Field Reading"=72063.72637333474}, {-0.373996, "Field Reading"=71675.853028433}, {-0.376007, "Field Reading"=71270.8145761266}, {-0.378006, "Field Reading"=70887.86580277358}, {-0.380014, "Field Reading"=70476.45894804779}, {-0.382015, "Field Reading"=70100.92669052206}, {-0.383981, "Field Reading"=69687.26293361597}, {-0.385979, "Field Reading"=69314.2188078024}, {-0.387997, "Field Reading"=68921.00490444242}, {-0.389992, "Field Reading"=68512.44141187714}, {-0.392002, "Field Reading"=68132.78873729035}, {-0.394008, "Field Reading"=67744.59773593211}, {-0.396009, "Field Reading"=67362.90429581849}, {-0.398009, "Field Reading"=66966.21311263024}, {-0.40002, "Field Reading"=66584.88232542733}, {-0.40202, "Field Reading"=66190.18688742137}, {-0.404029, "Field Reading"=65803.41175972404}, {-0.405987, "Field Reading"=65430.06333704008}, {-0.407992, "Field Reading"=65045.596581850645}, {-0.409994, "Field Reading"=64654.56609843408}, {-0.412001, "Field Reading"=64268.81145105208}, {-0.414003, "Field Reading"=63890.33781385515}, {-0.41601, "Field Reading"=63505.02685160026}, {-0.418015, "Field Reading"=63117.27765924839}, {-0.420025, "Field Reading"=62746.30192320907}, {-0.422024, "Field Reading"=62370.62894689783}, {-0.424028, "Field Reading"=61999.37712286325}, {-0.426028, "Field Reading"=61627.43600425867}, {-0.427994, "Field Reading"=61246.38133275711}, {-0.430001, "Field Reading"=60880.1838294113}, {-0.432007, "Field Reading"=60516.115656750306}, {-0.434006, "Field Reading"=60132.0392654017}, {-0.436012, "Field Reading"=59755.502562837486}, {-0.438009, "Field Reading"=59389.6818649604}, {-0.440016, "Field Reading"=59025.946325902594}, {-0.442016, "Field Reading"=58659.99930990735}, {-0.444021, "Field Reading"=58280.797779134096}, {-0.446023, "Field Reading"=57939.135868061465}, {-0.44803, "Field Reading"=57575.93281544165}, {-0.449998, "Field Reading"=57222.24200283823}, {-0.452002, "Field Reading"=56856.45569492873}, {-0.454003, "Field Reading"=56509.081223177025}, {-0.456008, "Field Reading"=56147.28059849981}, {-0.458016, "Field Reading"=55789.61472404594}, {-0.460012, "Field Reading"=55432.482587424376}, {-0.462015, "Field Reading"=55089.798225259874}, {-0.464016, "Field Reading"=54743.46374963279}, {-0.466018, "Field Reading"=54393.95106601023}, {-0.468027, "Field Reading"=54038.63539534256}, {-0.470028, "Field Reading"=53677.181818908546}, {-0.471994, "Field Reading"=53345.132703355484}, {-0.473999, "Field Reading"=52995.77709973849}, {-0.476006, "Field Reading"=52675.28420502821}, {-0.478008, "Field Reading"=52326.6926252344}, {-0.480011, "Field Reading"=51985.24952347946}, {-0.482016, "Field Reading"=51656.48931860708}, {-0.484016, "Field Reading"=51321.37570670591}, {-0.486025, "Field Reading"=50967.86777559771}, {-0.488023, "Field Reading"=50638.13494426955}, {-0.490024, "Field Reading"=50313.67499779246}, {-0.492028, "Field Reading"=49981.76582030953}, {-0.494033, "Field Reading"=49647.11699154548}, {-0.496014, "Field Reading"=49331.06575963719}, {-0.498009, "Field Reading"=49016.63385826772}, {-0.500013, "Field Reading"=48700.0350631136}, {-0.498004, "Field Reading"=49025.79247883442}, {-0.496006, "Field Reading"=49347.93855460045}, {-0.49403, "Field Reading"=49671.82391100637}, {-0.492022, "Field Reading"=50008.48683321188}, {-0.490024, "Field Reading"=50340.759430211605}, {-0.488019, "Field Reading"=50682.57843810267}, {-0.486018, "Field Reading"=51027.86900392249}, {-0.484006, "Field Reading"=51372.6081252627}, {-0.48201, "Field Reading"=51710.09903029484}, {-0.480006, "Field Reading"=52046.99351047161}, {-0.478006, "Field Reading"=52393.63567808351}, {-0.475996, "Field Reading"=52740.41966658024}, {-0.473993, "Field Reading"=53093.58723046765}, {-0.47199, "Field Reading"=53443.3776930315}, {-0.470021, "Field Reading"=53784.05408374376}, {-0.468024, "Field Reading"=54137.73877798419}, {-0.466013, "Field Reading"=54491.95272194913}, {-0.464014, "Field Reading"=54848.50920576081}, {-0.462008, "Field Reading"=55202.83704213504}, {-0.460009, "Field Reading"=55572.34774078665}, {-0.458008, "Field Reading"=55917.50724595216}, {-0.456002, "Field Reading"=56269.03390441217}, {-0.453998, "Field Reading"=56618.960201933536}, {-0.451999, "Field Reading"=56977.99157177667}, {-0.449997, "Field Reading"=57358.94703566986}, {-0.448026, "Field Reading"=57709.50361114295}, {-0.446018, "Field Reading"=58080.93238271967}, {-0.444018, "Field Reading"=58444.03026330338}, {-0.442013, "Field Reading"=58808.11953928785}, {-0.440015, "Field Reading"=59181.17564777641}, {-0.438011, "Field Reading"=59555.89819732358}, {-0.436011, "Field Reading"=59931.13591378931}, {-0.434004, "Field Reading"=60299.689473355145}, {-0.432005, "Field Reading"=60676.90483948897}, {-0.429998, "Field Reading"=61042.84375798529}, {-0.427987, "Field Reading"=61419.140966950334}, {-0.426018, "Field Reading"=61803.00471772018}, {-0.424016, "Field Reading"=62165.1419188365}, {-0.422013, "Field Reading"=62548.98531478067}, {-0.420016, "Field Reading"=62941.75561846161}, {-0.41801, "Field Reading"=63311.730110671706}, {-0.416011, "Field Reading"=63698.58504072161}, {-0.414001, "Field Reading"=64074.34463247107}, {-0.412005, "Field Reading"=64469.36255908968}, {-0.409998, "Field Reading"=64841.19365312322}, {-0.407997, "Field Reading"=65247.36609798692}, {-0.405994, "Field Reading"=65633.01227646456}, {-0.404031, "Field Reading"=66020.40266087561}, {-0.402021, "Field Reading"=66414.07508363276}, {-0.400021, "Field Reading"=66813.48158466577}, {-0.398012, "Field Reading"=67181.59752347064}, {-0.396014, "Field Reading"=67575.14482923374}, {-0.394009, "Field Reading"=67948.40178317367}, {-0.391997, "Field Reading"=68343.00080373378}, {-0.389995, "Field Reading"=68732.72847756816}, {-0.387993, "Field Reading"=69127.56939161295}, {-0.386003, "Field Reading"=69523.40813345509}, {-0.38398, "Field Reading"=69922.98965486472}, {-0.382012, "Field Reading"=70323.10796282934}, {-0.380008, "Field Reading"=70734.5629719804}, {-0.37801, "Field Reading"=71122.69280701425}, {-0.376007, "Field Reading"=71536.85316002458}, {-0.373993, "Field Reading"=71947.32741456095}, {-0.371995, "Field Reading"=72333.5867635535}, {-0.369989, "Field Reading"=72723.39522212744}, {-0.367993, "Field Reading"=73124.75160956998}, {-0.365987, "Field Reading"=73542.75678586643}, {-0.36398, "Field Reading"=73942.8536602708}, {-0.361978, "Field Reading"=74337.44267762493}, {-0.359975, "Field Reading"=74741.75966779134}, {-0.358009, "Field Reading"=75124.53992622033}, {-0.356007, "Field Reading"=75522.01444648331}, {-0.354001, "Field Reading"=75930.52162405061}, {-0.352004, "Field Reading"=76354.13164430657}, {-0.349996, "Field Reading"=76736.84879817758}, {-0.347993, "Field Reading"=77140.98241460565}, {-0.345985, "Field Reading"=77527.83056073425}, {-0.343982, "Field Reading"=77931.71103040628}, {-0.341982, "Field Reading"=78332.93248582719}, {-0.339976, "Field Reading"=78730.5880663792}, {-0.337977, "Field Reading"=79125.94992718982}, {-0.336009, "Field Reading"=79530.07505449794}, {-0.334004, "Field Reading"=79932.41723264841}, {-0.332005, "Field Reading"=80336.29427806102}, {-0.330001, "Field Reading"=80739.52285533234}, {-0.327996, "Field Reading"=81170.25172983836}, {-0.326, "Field Reading"=81530.16616147976}, {-0.323995, "Field Reading"=81950.60629208254}, {-0.321995, "Field Reading"=82341.76454492683}, {-0.319988, "Field Reading"=82753.73375573802}, {-0.317987, "Field Reading"=83137.5512114264}, {-0.315977, "Field Reading"=83534.56229726193}, {-0.314014, "Field Reading"=83917.20894186187}, {-0.31201, "Field Reading"=84316.08872362506}, {-0.310004, "Field Reading"=84722.53727060302}, {-0.308003, "Field Reading"=85143.67855810032}, {-0.306002, "Field Reading"=85546.14988929394}, {-0.304001, "Field Reading"=85941.29437340805}, {-0.301998, "Field Reading"=86332.5024013173}, {-0.299986, "Field Reading"=86721.70861302389}, {-0.297984, "Field Reading"=87126.25798943904}, {-0.295979, "Field Reading"=87539.52127864091}, {-0.293978, "Field Reading"=87928.90983920367}, {-0.29201, "Field Reading"=88308.05148304059}, {-0.290004, "Field Reading"=88711.4683992695}, {-0.288002, "Field Reading"=89108.15117340388}, {-0.285999, "Field Reading"=89511.47221848388}, {-0.283993, "Field Reading"=89898.79804876813}, {-0.281991, "Field Reading"=90298.37841992007}, {-0.279981, "Field Reading"=90678.28723001137}, {-0.27798, "Field Reading"=91101.85461326447}, {-0.275977, "Field Reading"=91460.03592425416}, {-0.273973, "Field Reading"=91860.18440905282}, {-0.271975, "Field Reading"=92239.31519578917}, {-0.269975, "Field Reading"=92633.89410622318}, {-0.268002, "Field Reading"=93014.26439454414}, {-0.266006, "Field Reading"=93413.77506048934}, {-0.263996, "Field Reading"=93844.89053040941}, {-0.261996, "Field Reading"=94182.18419728233}, {-0.259994, "Field Reading"=94568.72031019257}, {-0.25799, "Field Reading"=94944.20891479714}, {-0.255981, "Field Reading"=95336.36495681612}, {-0.253979, "Field Reading"=95716.52000226121}, {-0.251976, "Field Reading"=96099.953470988}, {-0.249978, "Field Reading"=96496.85585575154}, {-0.247975, "Field Reading"=96867.88310617869}, {-0.245998, "Field Reading"=97237.02309990987}, {-0.243995, "Field Reading"=97620.25741869146}, {-0.241994, "Field Reading"=98019.3127136631}, {-0.239988, "Field Reading"=98369.04171465813}, {-0.237987, "Field Reading"=98771.92399956836}, {-0.235979, "Field Reading"=99142.09250444289}, {-0.23398, "Field Reading"=99510.48564417282}, {-0.231977, "Field Reading"=99884.17453906633}, {-0.229973, "Field Reading"=100244.53821073005}, {-0.227966, "Field Reading"=100648.12934330545}, {-0.225965, "Field Reading"=100998.52054476134}, {-0.224, "Field Reading"=101441.46510458887}, {-0.221994, "Field Reading"=101724.78577647437}, {-0.219993, "Field Reading"=102099.60597580162}, {-0.217984, "Field Reading"=102460.64611349524}, {-0.215986, "Field Reading"=102838.23354362577}, {-0.213981, "Field Reading"=103173.09546769528}, {-0.21198, "Field Reading"=103554.9063765553}, {-0.20997, "Field Reading"=103901.82349011555}, {-0.207967, "Field Reading"=104291.68192007384}, {-0.205961, "Field Reading"=104731.61256203726}, {-0.20396, "Field Reading"=105076.60762676063}, {-0.20199, "Field Reading"=105349.07736760304}, {-0.199959, "Field Reading"=105732.39987732527}, {-0.19796, "Field Reading"=106084.47745517294}, {-0.195959, "Field Reading"=106429.46757838596}, {-0.193956, "Field Reading"=106771.03976747258}, {-0.191961, "Field Reading"=107116.90949572282}, {-0.18996, "Field Reading"=107481.13026061174}, {-0.187961, "Field Reading"=107855.5812498924}, {-0.185959, "Field Reading"=108174.81646946588}, {-0.183961, "Field Reading"=108542.44968521917}, {-0.181961, "Field Reading"=108884.3543928097}, {-0.179962, "Field Reading"=109240.67767802403}, {-0.177968, "Field Reading"=109576.76062408411}, {-0.175967, "Field Reading"=109916.85978599671}, {-0.173965, "Field Reading"=110247.47298710352}, {-0.171965, "Field Reading"=110591.98044953214}, {-0.169964, "Field Reading"=110928.80125832958}, {-0.167962, "Field Reading"=111261.84908685024}, {-0.165963, "Field Reading"=111626.5461369277}, {-0.163964, "Field Reading"=111959.0303857972}, {-0.161966, "Field Reading"=112264.33403571032}, {-0.159966, "Field Reading"=112626.73200405543}, {-0.157964, "Field Reading"=112925.80227761771}, {-0.155961, "Field Reading"=113255.68053911565}, {-0.15396, "Field Reading"=113586.7319837101}, {-0.151961, "Field Reading"=113895.00981847073}, {-0.149963, "Field Reading"=114222.71307791912}, {-0.147966, "Field Reading"=114544.27224449984}, {-0.145965, "Field Reading"=114964.75406608121}, {-0.143965, "Field Reading"=115291.90357972292}, {-0.141965, "Field Reading"=115601.97060380278}, {-0.139967, "Field Reading"=115932.94182935619}, {-0.137966, "Field Reading"=116148.63954741381}, {-0.135962, "Field Reading"=116467.64549675342}, {-0.133963, "Field Reading"=116759.63533041644}, {-0.131967, "Field Reading"=117093.75166367943}, {-0.129969, "Field Reading"=117405.44349192872}, {-0.127968, "Field Reading"=117703.11163436687}, {-0.125967, "Field Reading"=118009.61187150446}, {-0.123964, "Field Reading"=118313.35420325267}, {-0.121962, "Field Reading"=118630.84584857209}, {-0.119961, "Field Reading"=118918.08836503861}, {-0.117965, "Field Reading"=119213.76417978322}, {-0.115963, "Field Reading"=119510.67436863286}, {-0.113966, "Field Reading"=119800.52517717896}, {-0.111967, "Field Reading"=120114.74338825553}, {-0.109966, "Field Reading"=120393.12846305688}, {-0.107968, "Field Reading"=120670.50095335596}, {-0.105968, "Field Reading"=120950.0873158093}, {-0.103971, "Field Reading"=121240.49629180465}, {-0.101971, "Field Reading"=121520.9212475406}, {-0.0999734, "Field Reading"=121793.42237989193}, {-0.0979708, "Field Reading"=122061.91629538818}, {-0.0959695, "Field Reading"=122339.69999400855}, {-0.0939698, "Field Reading"=122678.54158833605}, {-0.0919739, "Field Reading"=122881.06947556311}, {-0.0899753, "Field Reading"=123140.81596343082}, {-0.0879776, "Field Reading"=123396.28146003748}, {-0.0859743, "Field Reading"=123654.56695019835}, {-0.0839735, "Field Reading"=123911.74109619767}, {-0.0819712, "Field Reading"=124161.53941696278}, {-0.0799742, "Field Reading"=124402.98414594689}, {-0.0779748, "Field Reading"=124653.57487706463}, {-0.0759753, "Field Reading"=124900.82773699828}, {-0.0739803, "Field Reading"=125154.87811067313}, {-0.0719775, "Field Reading"=125391.75396022097}, {-0.0699769, "Field Reading"=125616.89279187743}, {-0.067973, "Field Reading"=125836.54374834543}, {-0.0659737, "Field Reading"=126064.2343130773}, {-0.0639725, "Field Reading"=126296.07840040434}, {-0.0619723, "Field Reading"=126491.89375646776}, {-0.0599715, "Field Reading"=126707.40132725693}, {-0.0579734, "Field Reading"=126915.88621367555}, {-0.0559742, "Field Reading"=127108.3598642947}, {-0.0539768, "Field Reading"=127312.78156473335}, {-0.0519753, "Field Reading"=127496.37566507467}, {-0.0499765, "Field Reading"=127695.64506403115}, {-0.0479753, "Field Reading"=127885.36638028699}, {-0.0459754, "Field Reading"=128071.60247589015}, {-0.0439772, "Field Reading"=128244.0700109064}, {-0.0419794, "Field Reading"=128417.03400744572}, {-0.0399775, "Field Reading"=128576.02315670981}, {-0.0379795, "Field Reading"=128738.8309628083}, {-0.0359774, "Field Reading"=128888.88888888888}, {-0.0339733, "Field Reading"=129045.52809705773}, {-0.0319713, "Field Reading"=129204.63776081344}, {-0.0299684, "Field Reading"=129338.59864914439}, {-0.0279702, "Field Reading"=129479.67780761041}, {-0.0259681, "Field Reading"=129600.091829656}, {-0.0239672, "Field Reading"=129731.25118406452}, {-0.0219603, "Field Reading"=129824.30211523226}, {-0.0199614, "Field Reading"=129946.03321333483}, {-0.0179615, "Field Reading"=130054.01569785962}, {-0.0159585, "Field Reading"=130139.61150163913}, {-0.0139637, "Field Reading"=130211.0239744869}, {-0.0119623, "Field Reading"=130254.7864330226}, {-0.00996189, "Field Reading"=130248.02573087181}, {-0.00796263, "Field Reading"=130307.20085882704}, {-0.00595863, "Field Reading"=130224.77680766668}, {-0.00395613, "Field Reading"=130013.11262065092}, {-0.00195336, "Field Reading"=129228.0822461563}]
  in  "Wait (ms)":u32=100
  out "Voltage (V)":dbl=-0.00195336 format="%#_13g"
  in  "Set Compliance current (A)":dbl=0.0001 min=0.0 step=0.1 format="%_3f"
  out "Current (A)":dbl=-1.51156e-08
  in  "Folder":path=path "D:/Pranava/Data/STS/MA1981"
  out "I vs V":cluster{dbl, "Field Reading":dbl}[](graph)=[{9.24826e-05, "Field Reading"=2.87887e-10}, {0.00208223, "Field Reading"=1.56063e-08}, {0.00408287, "Field Reading"=3.08768e-08}, {0.00608664, "Field Reading"=4.61809e-08}, {0.00808966, "Field Reading"=6.14589e-08}, {0.0100896, "Field Reading"=7.67114e-08}, {0.0120913, "Field Reading"=9.19816e-08}, {0.0140768, "Field Reading"=1.07045e-07}, {0.0160766, "Field Reading"=1.22619e-07}, {0.0180795, "Field Reading"=1.37946e-07}, {0.0200782, "Field Reading"=1.53241e-07}, {0.0220798, "Field Reading"=1.68579e-07}, {0.0240771, "Field Reading"=1.83876e-07}, {0.0260761, "Field Reading"=1.99226e-07}, {0.0280696, "Field Reading"=2.14461e-07}, {0.0300689, "Field Reading"=2.29837e-07}, {0.0320729, "Field Reading"=2.45184e-07}, {0.0340708, "Field Reading"=2.60562e-07}, {0.0360752, "Field Reading"=2.7598e-07}, {0.0380763, "Field Reading"=2.914e-07}, {0.0400745, "Field Reading"=3.06857e-07}, {0.042069, "Field Reading"=3.22306e-07}, {0.0440687, "Field Reading"=3.37789e-07}, {0.0460705, "Field Reading"=3.53329e-07}, {0.0480758, "Field Reading"=3.68941e-07}, {0.0500756, "Field Reading"=3.84549e-07}, {0.0520796, "Field Reading"=4.00195e-07}, {0.0540786, "Field Reading"=4.15897e-07}, {0.0560762, "Field Reading"=4.31665e-07}, {0.0580758, "Field Reading"=4.47391e-07}, {0.0600795, "Field Reading"=4.63197e-07}, {0.06208, "Field Reading"=4.79108e-07}, {0.0640783, "Field Reading"=4.94929e-07}, {0.0660839, "Field Reading"=5.10914e-07}, {0.0680779, "Field Reading"=5.26898e-07}, {0.0700804, "Field Reading"=5.4302e-07}, {0.0720784, "Field Reading"=5.58967e-07}, {0.0740798, "Field Reading"=5.75255e-07}, {0.0760786, "Field Reading"=5.91498e-07}, {0.0780784, "Field Reading"=6.07691e-07}, {0.080081, "Field Reading"=6.24109e-07}, {0.082076, "Field Reading"=6.40444e-07}, {0.0840742, "Field Reading"=6.56928e-07}, {0.0860755, "Field Reading"=6.73444e-07}, {0.0880753, "Field Reading"=6.89988e-07}, {0.0900754, "Field Reading"=7.06611e-07}, {0.0920787, "Field Reading"=7.23346e-07}, {0.094079, "Field Reading"=7.40218e-07}, {0.0960754, "Field Reading"=7.56919e-07}, {0.0980756, "Field Reading"=7.73915e-07}, {0.100075, "Field Reading"=7.90827e-07}, {0.102075, "Field Reading"=8.07935e-07}, {0.104078, "Field Reading"=8.25279e-07}, {0.106077, "Field Reading"=8.42372e-07}, {0.108078, "Field Reading"=8.59801e-07}, {0.110074, "Field Reading"=8.77114e-07}, {0.112071, "Field Reading"=8.94482e-07}, {0.114072, "Field Reading"=9.12143e-07}, {0.116073, "Field Reading"=9.29871e-07}, {0.118074, "Field Reading"=9.47471e-07}, {0.120074, "Field Reading"=9.65385e-07}, {0.122073, "Field Reading"=9.83248e-07}, {0.124068, "Field Reading"=1.00129e-06}, {0.12607, "Field Reading"=1.01931e-06}, {0.12807, "Field Reading"=1.03755e-06}, {0.130073, "Field Reading"=1.05584e-06}, {0.13207, "Field Reading"=1.07419e-06}, {0.134072, "Field Reading"=1.09274e-06}, {0.136065, "Field Reading"=1.11143e-06}, {0.138062, "Field Reading"=1.12991e-06}, {0.140062, "Field Reading"=1.14919e-06}, {0.142063, "Field Reading"=1.16796e-06}, {0.144064, "Field Reading"=1.18703e-06}, {0.146064, "Field Reading"=1.20629e-06}, {0.148066, "Field Reading"=1.22537e-06}, {0.150064, "Field Reading"=1.24453e-06}, {0.152064, "Field Reading"=1.26384e-06}, {0.154064, "Field Reading"=1.28353e-06}, {0.156068, "Field Reading"=1.30333e-06}, {0.158069, "Field Reading"=1.32303e-06}, {0.160068, "Field Reading"=1.34303e-06}, {0.162069, "Field Reading"=1.36313e-06}, {0.164067, "Field Reading"=1.38334e-06}, {0.166065, "Field Reading"=1.40356e-06}, {0.168064, "Field Reading"=1.42387e-06}, {0.170065, "Field Reading"=1.44468e-06}, {0.172066, "Field Reading"=1.46544e-06}, {0.174067, "Field Reading"=1.48628e-06}, {0.176067, "Field Reading"=1.50722e-06}, {0.178062, "Field Reading"=1.52821e-06}, {0.180063, "Field Reading"=1.54954e-06}, {0.182065, "Field Reading"=1.57082e-06}, {0.184064, "Field Reading"=1.59239e-06}, {0.186063, "Field Reading"=1.61402e-06}, {0.188066, "Field Reading"=1.63606e-06}, {0.190068, "Field Reading"=1.65818e-06}, {0.192063, "Field Reading"=1.68023e-06}, {0.194061, "Field Reading"=1.70245e-06}, {0.196063, "Field Reading"=1.72505e-06}, {0.198066, "Field Reading"=1.7477e-06}, {0.200067, "Field Reading"=1.77039e-06}, {0.202094, "Field Reading"=1.79383e-06}, {0.2041, "Field Reading"=1.8172e-06}, {0.206103, "Field Reading"=1.84065e-06}, {0.20811, "Field Reading"=1.86391e-06}, {0.210077, "Field Reading"=1.88743e-06}, {0.212084, "Field Reading"=1.91084e-06}, {0.214085, "Field Reading"=1.9352e-06}, {0.216093, "Field Reading"=1.95972e-06}, {0.218084, "Field Reading"=1.98412e-06}, {0.220093, "Field Reading"=2.00875e-06}, {0.222097, "Field Reading"=2.03381e-06}, {0.224105, "Field Reading"=2.05876e-06}, {0.226104, "Field Reading"=2.08362e-06}, {0.228108, "Field Reading"=2.10935e-06}, {0.23008, "Field Reading"=2.13426e-06}, {0.232083, "Field Reading"=2.16017e-06}, {0.234082, "Field Reading"=2.18645e-06}, {0.236089, "Field Reading"=2.2126e-06}, {0.238094, "Field Reading"=2.23936e-06}, {0.240097, "Field Reading"=2.26598e-06}, {0.242102, "Field Reading"=2.29305e-06}, {0.244106, "Field Reading"=2.31986e-06}, {0.246111, "Field Reading"=2.3476e-06}, {0.248119, "Field Reading"=2.37579e-06}, {0.250125, "Field Reading"=2.40297e-06}, {0.252088, "Field Reading"=2.43029e-06}, {0.254094, "Field Reading"=2.45893e-06}, {0.256097, "Field Reading"=2.48761e-06}, {0.258105, "Field Reading"=2.51683e-06}, {0.260109, "Field Reading"=2.54583e-06}, {0.262107, "Field Reading"=2.57546e-06}, {0.264109, "Field Reading"=2.60511e-06}, {0.266118, "Field Reading"=2.63503e-06}, {0.268115, "Field Reading"=2.66528e-06}, {0.27012, "Field Reading"=2.69574e-06}, {0.272085, "Field Reading"=2.72543e-06}, {0.274093, "Field Reading"=2.75668e-06}, {0.276096, "Field Reading"=2.78829e-06}, {0.2781, "Field Reading"=2.81972e-06}, {0.280098, "Field Reading"=2.85176e-06}, {0.282103, "Field Reading"=2.88397e-06}, {0.284104, "Field Reading"=2.91606e-06}, {0.28611, "Field Reading"=2.94977e-06}, {0.288119, "Field Reading"=2.98267e-06}, {0.29012, "Field Reading"=3.01543e-06}, {0.292129, "Field Reading"=3.04957e-06}, {0.294094, "Field Reading"=3.08345e-06}, {0.296091, "Field Reading"=3.11753e-06}, {0.298098, "Field Reading"=3.15239e-06}, {0.300094, "Field Reading"=3.18769e-06}, {0.302104, "Field Reading"=3.22287e-06}, {0.304106, "Field Reading"=3.25853e-06}, {0.306113, "Field Reading"=3.29506e-06}, {0.308113, "Field Reading"=3.33209e-06}, {0.310119, "Field Reading"=3.36914e-06}, {0.312124, "Field Reading"=3.40592e-06}, {0.314088, "Field Reading"=3.44326e-06}, {0.316094, "Field Reading"=3.48104e-06}, {0.318097, "Field Reading"=3.51853e-06}, {0.320102, "Field Reading"=3.55754e-06}, {0.322106, "Field Reading"=3.59716e-06}, {0.324107, "Field Reading"=3.6366e-06}, {0.326113, "Field Reading"=3.67698e-06}, {0.328116, "Field Reading"=3.71654e-06}, {0.33012, "Field Reading"=3.75777e-06}, {0.332121, "Field Reading"=3.79827e-06}, {0.334123, "Field Reading"=3.83984e-06}, {0.33609, "Field Reading"=3.88072e-06}, {0.338095, "Field Reading"=3.92289e-06}, {0.340103, "Field Reading"=3.96586e-06}, {0.342109, "Field Reading"=4.00893e-06}, {0.34411, "Field Reading"=4.05259e-06}, {0.346114, "Field Reading"=4.09781e-06}, {0.348119, "Field Reading"=4.14284e-06}, {0.350126, "Field Reading"=4.18804e-06}, {0.352124, "Field Reading"=4.23333e-06}, {0.354127, "Field Reading"=4.27975e-06}, {0.356091, "Field Reading"=4.32583e-06}, {0.358103, "Field Reading"=4.37286e-06}, {0.360106, "Field Reading"=4.42088e-06}, {0.362108, "Field Reading"=4.46855e-06}, {0.364112, "Field Reading"=4.51755e-06}, {0.366113, "Field Reading"=4.56709e-06}, {0.368121, "Field Reading"=4.61641e-06}, {0.370123, "Field Reading"=4.66597e-06}, {0.372125, "Field Reading"=4.7161e-06}, {0.374122, "Field Reading"=4.76726e-06}, {0.376098, "Field Reading"=4.81914e-06}, {0.378101, "Field Reading"=4.86966e-06}, {0.380109, "Field Reading"=4.92386e-06}, {0.382109, "Field Reading"=4.97615e-06}, {0.384122, "Field Reading"=5.03166e-06}, {0.386122, "Field Reading"=5.08606e-06}, {0.388125, "Field Reading"=5.14195e-06}, {0.39013, "Field Reading"=5.19672e-06}, {0.392133, "Field Reading"=5.25434e-06}, {0.394136, "Field Reading"=5.31058e-06}, {0.39614, "Field Reading"=5.36809e-06}, {0.398104, "Field Reading"=5.42457e-06}, {0.400107, "Field Reading"=5.48326e-06}, {0.40211, "Field Reading"=5.54257e-06}, {0.40412, "Field Reading"=5.6026e-06}, {0.40612, "Field Reading"=5.66328e-06}, {0.408124, "Field Reading"=5.72501e-06}, {0.410125, "Field Reading"=5.78689e-06}, {0.412135, "Field Reading"=5.84873e-06}, {0.414137, "Field Reading"=5.91407e-06}, {0.416143, "Field Reading"=5.97804e-06}, {0.418111, "Field Reading"=6.04122e-06}, {0.420117, "Field Reading"=6.10642e-06}, {0.422119, "Field Reading"=6.17456e-06}, {0.42412, "Field Reading"=6.2407e-06}, {0.426121, "Field Reading"=6.3069e-06}, {0.428125, "Field Reading"=6.37553e-06}, {0.430128, "Field Reading"=6.44545e-06}, {0.432133, "Field Reading"=6.51454e-06}, {0.434134, "Field Reading"=6.58404e-06}, {0.436139, "Field Reading"=6.6544e-06}, {0.438137, "Field Reading"=6.72643e-06}, {0.440108, "Field Reading"=6.79777e-06}, {0.44211, "Field Reading"=6.87118e-06}, {0.44411, "Field Reading"=6.94645e-06}, {0.446114, "Field Reading"=7.02217e-06}, {0.448117, "Field Reading"=7.09667e-06}, {0.450123, "Field Reading"=7.17352e-06}, {0.452128, "Field Reading"=7.253e-06}, {0.45413, "Field Reading"=7.3321e-06}, {0.456133, "Field Reading"=7.41066e-06}, {0.458137, "Field Reading"=7.49013e-06}, {0.460102, "Field Reading"=7.57094e-06}, {0.4621, "Field Reading"=7.65338e-06}, {0.464111, "Field Reading"=7.73533e-06}, {0.466115, "Field Reading"=7.81743e-06}, {0.468126, "Field Reading"=7.90206e-06}, {0.470129, "Field Reading"=7.98872e-06}, {0.472136, "Field Reading"=8.07598e-06}, {0.474135, "Field Reading"=8.16016e-06}, {0.476139, "Field Reading"=8.24866e-06}, {0.478142, "Field Reading"=8.33775e-06}, {0.480145, "Field Reading"=8.42615e-06}, {0.482113, "Field Reading"=8.51446e-06}, {0.484118, "Field Reading"=8.60652e-06}, {0.486126, "Field Reading"=8.69921e-06}, {0.488123, "Field Reading"=8.79344e-06}, {0.490129, "Field Reading"=8.88506e-06}, {0.49213, "Field Reading"=8.98057e-06}, {0.494141, "Field Reading"=9.07809e-06}, {0.49614, "Field Reading"=9.17364e-06}, {0.498144, "Field Reading"=9.27348e-06}, {0.500151, "Field Reading"=9.37278e-06}, {0.498148, "Field Reading"=9.27752e-06}, {0.496145, "Field Reading"=9.1772e-06}, {0.494146, "Field Reading"=9.08009e-06}, {0.492136, "Field Reading"=8.9814e-06}, {0.490135, "Field Reading"=8.88787e-06}, {0.488125, "Field Reading"=8.79329e-06}, {0.486143, "Field Reading"=8.70173e-06}, {0.484113, "Field Reading"=8.60723e-06}, {0.48212, "Field Reading"=8.51757e-06}, {0.480148, "Field Reading"=8.42826e-06}, {0.478147, "Field Reading"=8.33798e-06}, {0.476143, "Field Reading"=8.25164e-06}, {0.47414, "Field Reading"=8.16547e-06}, {0.472135, "Field Reading"=8.08159e-06}, {0.470131, "Field Reading"=7.99569e-06}, {0.46813, "Field Reading"=7.90814e-06}, {0.466119, "Field Reading"=7.82404e-06}, {0.464119, "Field Reading"=7.74139e-06}, {0.462114, "Field Reading"=7.65806e-06}, {0.460119, "Field Reading"=7.57421e-06}, {0.458148, "Field Reading"=7.49583e-06}, {0.456138, "Field Reading"=7.41431e-06}, {0.454138, "Field Reading"=7.33799e-06}, {0.452139, "Field Reading"=7.2587e-06}, {0.450134, "Field Reading"=7.18319e-06}, {0.448129, "Field Reading"=7.10721e-06}, {0.446123, "Field Reading"=7.03424e-06}, {0.444124, "Field Reading"=6.9594e-06}, {0.442118, "Field Reading"=6.88454e-06}, {0.440114, "Field Reading"=6.81194e-06}, {0.438145, "Field Reading"=6.73898e-06}, {0.436145, "Field Reading"=6.66651e-06}, {0.43414, "Field Reading"=6.59749e-06}, {0.432137, "Field Reading"=6.5262e-06}, {0.430135, "Field Reading"=6.45725e-06}, {0.428127, "Field Reading"=6.38839e-06}, {0.426126, "Field Reading"=6.32049e-06}, {0.424124, "Field Reading"=6.25312e-06}, {0.422123, "Field Reading"=6.18644e-06}, {0.420119, "Field Reading"=6.11952e-06}, {0.418111, "Field Reading"=6.0543e-06}, {0.416145, "Field Reading"=5.99008e-06}, {0.414139, "Field Reading"=5.92611e-06}, {0.41214, "Field Reading"=5.86396e-06}, {0.410131, "Field Reading"=5.80023e-06}, {0.408128, "Field Reading"=5.73756e-06}, {0.406125, "Field Reading"=5.67868e-06}, {0.404124, "Field Reading"=5.61838e-06}, {0.40212, "Field Reading"=5.55772e-06}, {0.400116, "Field Reading"=5.49844e-06}, {0.398111, "Field Reading"=5.4392e-06}, {0.396139, "Field Reading"=5.38207e-06}, {0.394134, "Field Reading"=5.32433e-06}, {0.392128, "Field Reading"=5.26861e-06}, {0.390125, "Field Reading"=5.21211e-06}, {0.388125, "Field Reading"=5.15583e-06}, {0.38612, "Field Reading"=5.10211e-06}, {0.384116, "Field Reading"=5.04776e-06}, {0.382109, "Field Reading"=4.99309e-06}, {0.380107, "Field Reading"=4.9392e-06}, {0.378106, "Field Reading"=4.88722e-06}, {0.376101, "Field Reading"=4.83529e-06}, {0.37413, "Field Reading"=4.78309e-06}, {0.372128, "Field Reading"=4.73125e-06}, {0.370126, "Field Reading"=4.68108e-06}, {0.368119, "Field Reading"=4.6315e-06}, {0.366114, "Field Reading"=4.58221e-06}, {0.364111, "Field Reading"=4.53334e-06}, {0.36211, "Field Reading"=4.48395e-06}, {0.360107, "Field Reading"=4.43568e-06}, {0.358103, "Field Reading"=4.38801e-06}, {0.356093, "Field Reading"=4.3405e-06}, {0.354124, "Field Reading"=4.29388e-06}, {0.352115, "Field Reading"=4.24792e-06}, {0.350114, "Field Reading"=4.20357e-06}, {0.34811, "Field Reading"=4.1573e-06}, {0.346107, "Field Reading"=4.11321e-06}, {0.344101, "Field Reading"=4.06839e-06}, {0.3421, "Field Reading"=4.02446e-06}, {0.340095, "Field Reading"=3.98127e-06}, {0.338091, "Field Reading"=3.93772e-06}, {0.336087, "Field Reading"=3.8958e-06}, {0.334123, "Field Reading"=3.85487e-06}, {0.332117, "Field Reading"=3.81271e-06}, {0.330117, "Field Reading"=3.77094e-06}, {0.328107, "Field Reading"=3.73036e-06}, {0.326111, "Field Reading"=3.68919e-06}, {0.324107, "Field Reading"=3.65069e-06}, {0.322109, "Field Reading"=3.61117e-06}, {0.320099, "Field Reading"=3.57229e-06}, {0.318093, "Field Reading"=3.53327e-06}, {0.316093, "Field Reading"=3.49532e-06}, {0.314091, "Field Reading"=3.45906e-06}, {0.31212, "Field Reading"=3.42149e-06}, {0.310117, "Field Reading"=3.38256e-06}, {0.308112, "Field Reading"=3.34647e-06}, {0.306114, "Field Reading"=3.30967e-06}, {0.304108, "Field Reading"=3.27349e-06}, {0.302107, "Field Reading"=3.23776e-06}, {0.300098, "Field Reading"=3.20212e-06}, {0.298095, "Field Reading"=3.16679e-06}, {0.296094, "Field Reading"=3.13176e-06}, {0.294092, "Field Reading"=3.09697e-06}, {0.29212, "Field Reading"=3.06395e-06}, {0.290125, "Field Reading"=3.02974e-06}, {0.28812, "Field Reading"=2.9961e-06}, {0.286114, "Field Reading"=2.96265e-06}, {0.284114, "Field Reading"=2.92954e-06}, {0.282104, "Field Reading"=2.89684e-06}, {0.280102, "Field Reading"=2.86475e-06}, {0.2781, "Field Reading"=2.83259e-06}, {0.276096, "Field Reading"=2.80106e-06}, {0.274095, "Field Reading"=2.76977e-06}, {0.272086, "Field Reading"=2.73867e-06}, {0.270118, "Field Reading"=2.70818e-06}, {0.268115, "Field Reading"=2.67738e-06}, {0.266113, "Field Reading"=2.64691e-06}, {0.264107, "Field Reading"=2.61697e-06}, {0.262103, "Field Reading"=2.58743e-06}, {0.260103, "Field Reading"=2.55782e-06}, {0.258096, "Field Reading"=2.5284e-06}, {0.256092, "Field Reading"=2.49936e-06}, {0.254086, "Field Reading"=2.47049e-06}, {0.252086, "Field Reading"=2.44219e-06}, {0.250122, "Field Reading"=2.4144e-06}, {0.248116, "Field Reading"=2.38659e-06}, {0.24611, "Field Reading"=2.35881e-06}, {0.244101, "Field Reading"=2.33097e-06}, {0.242097, "Field Reading"=2.30406e-06}, {0.240094, "Field Reading"=2.27665e-06}, {0.238089, "Field Reading"=2.24988e-06}, {0.236082, "Field Reading"=2.22309e-06}, {0.23408, "Field Reading"=2.19713e-06}, {0.232076, "Field Reading"=2.17118e-06}, {0.230075, "Field Reading"=2.14527e-06}, {0.228099, "Field Reading"=2.11966e-06}, {0.226096, "Field Reading"=2.09411e-06}, {0.224093, "Field Reading"=2.06858e-06}, {0.222093, "Field Reading"=2.04389e-06}, {0.220095, "Field Reading"=2.01883e-06}, {0.21809, "Field Reading"=1.99438e-06}, {0.216086, "Field Reading"=1.96941e-06}, {0.214077, "Field Reading"=1.9452e-06}, {0.212077, "Field Reading"=1.92109e-06}, {0.210073, "Field Reading"=1.89708e-06}, {0.208101, "Field Reading"=1.87374e-06}, {0.206095, "Field Reading"=1.84988e-06}, {0.204095, "Field Reading"=1.82672e-06}, {0.202089, "Field Reading"=1.8032e-06}, {0.200064, "Field Reading"=1.77961e-06}, {0.198062, "Field Reading"=1.75666e-06}, {0.196061, "Field Reading"=1.73406e-06}, {0.194063, "Field Reading"=1.71129e-06}, {0.192065, "Field Reading"=1.68874e-06}, {0.190067, "Field Reading"=1.6668e-06}, {0.188066, "Field Reading"=1.64463e-06}, {0.186066, "Field Reading"=1.62268e-06}, {0.184067, "Field Reading"=1.60081e-06}, {0.182063, "Field Reading"=1.57885e-06}, {0.180062, "Field Reading"=1.55763e-06}, {0.178062, "Field Reading"=1.53626e-06}, {0.176065, "Field Reading"=1.51494e-06}, {0.174063, "Field Reading"=1.49385e-06}, {0.17206, "Field Reading"=1.47285e-06}, {0.17006, "Field Reading"=1.45197e-06}, {0.16806, "Field Reading"=1.43108e-06}, {0.166061, "Field Reading"=1.4109e-06}, {0.164059, "Field Reading"=1.39053e-06}, {0.162066, "Field Reading"=1.37005e-06}, {0.160064, "Field Reading"=1.34989e-06}, {0.158063, "Field Reading"=1.32975e-06}, {0.156057, "Field Reading"=1.30993e-06}, {0.154056, "Field Reading"=1.28998e-06}, {0.152056, "Field Reading"=1.27042e-06}, {0.150057, "Field Reading"=1.25053e-06}, {0.148063, "Field Reading"=1.23112e-06}, {0.146063, "Field Reading"=1.2119e-06}, {0.144062, "Field Reading"=1.19256e-06}, {0.142062, "Field Reading"=1.17355e-06}, {0.140061, "Field Reading"=1.15443e-06}, {0.138061, "Field Reading"=1.13546e-06}, {0.136064, "Field Reading"=1.11666e-06}, {0.134067, "Field Reading"=1.09801e-06}, {0.132062, "Field Reading"=1.07939e-06}, {0.130064, "Field Reading"=1.06076e-06}, {0.128063, "Field Reading"=1.04243e-06}, {0.126063, "Field Reading"=1.02422e-06}, {0.124066, "Field Reading"=1.00606e-06}, {0.122069, "Field Reading"=9.87995e-07}, {0.120073, "Field Reading"=9.70021e-07}, {0.118072, "Field Reading"=9.52161e-07}, {0.116074, "Field Reading"=9.34236e-07}, {0.114072, "Field Reading"=9.16335e-07}, {0.112071, "Field Reading"=8.98615e-07}, {0.110071, "Field Reading"=8.81175e-07}, {0.108072, "Field Reading"=8.63613e-07}, {0.106072, "Field Reading"=8.46207e-07}, {0.104071, "Field Reading"=8.28883e-07}, {0.10207, "Field Reading"=8.11538e-07}, {0.100074, "Field Reading"=7.94407e-07}, {0.0980714, "Field Reading"=7.77317e-07}, {0.0960723, "Field Reading"=7.60392e-07}, {0.0940741, "Field Reading"=7.43375e-07}, {0.0920758, "Field Reading"=7.2646e-07}, {0.0900749, "Field Reading"=7.09738e-07}, {0.0880718, "Field Reading"=6.92925e-07}, {0.0860697, "Field Reading"=6.76231e-07}, {0.0840724, "Field Reading"=6.59525e-07}, {0.0820718, "Field Reading"=6.43072e-07}, {0.0800771, "Field Reading"=6.26698e-07}, {0.078074, "Field Reading"=6.10314e-07}, {0.0760751, "Field Reading"=5.93936e-07}, {0.0740699, "Field Reading"=5.77557e-07}, {0.0720729, "Field Reading"=5.61342e-07}, {0.0700725, "Field Reading"=5.45212e-07}, {0.0680684, "Field Reading"=5.29041e-07}, {0.066073, "Field Reading"=5.13012e-07}, {0.0640697, "Field Reading"=4.96969e-07}, {0.0620658, "Field Reading"=4.80912e-07}, {0.0600666, "Field Reading"=4.65011e-07}, {0.0580685, "Field Reading"=4.49108e-07}, {0.0560677, "Field Reading"=4.33278e-07}, {0.054073, "Field Reading"=4.17476e-07}, {0.0520688, "Field Reading"=4.01714e-07}, {0.0500681, "Field Reading"=3.85963e-07}, {0.0480689, "Field Reading"=3.70322e-07}, {0.0460666, "Field Reading"=3.54681e-07}, {0.0440633, "Field Reading"=3.39043e-07}, {0.042061, "Field Reading"=3.23476e-07}, {0.0400637, "Field Reading"=3.07953e-07}, {0.0380634, "Field Reading"=2.92371e-07}, {0.0360641, "Field Reading"=2.76911e-07}, {0.0340635, "Field Reading"=2.61464e-07}, {0.0320607, "Field Reading"=2.45999e-07}, {0.0300555, "Field Reading"=2.30557e-07}, {0.0280551, "Field Reading"=2.15141e-07}, {0.026058, "Field Reading"=1.99831e-07}, {0.0240593, "Field Reading"=1.84446e-07}, {0.0220574, "Field Reading"=1.69046e-07}, {0.0200566, "Field Reading"=1.53705e-07}, {0.01806, "Field Reading"=1.38382e-07}, {0.0160547, "Field Reading"=1.23021e-07}, {0.0140561, "Field Reading"=1.07676e-07}, {0.012063, "Field Reading"=9.21916e-08}, {0.0100592, "Field Reading"=7.69104e-08}, {0.00805471, "Field Reading"=6.15975e-08}, {0.00605381, "Field Reading"=4.63368e-08}, {0.00404904, "Field Reading"=3.09935e-08}, {0.00205326, "Field Reading"=1.56838e-08}, {4.89712e-05, "Field Reading"=2.85623e-10}, {-0.00196376, "Field Reading"=-1.55605e-08}, {-0.0039638, "Field Reading"=-3.08585e-08}, {-0.00596104, "Field Reading"=-4.61845e-08}, {-0.0079607, "Field Reading"=-6.15323e-08}, {-0.00995808, "Field Reading"=-7.68695e-08}, {-0.0119533, "Field Reading"=-9.22288e-08}, {-0.0139638, "Field Reading"=-1.07624e-07}, {-0.0159607, "Field Reading"=-1.23407e-07}, {-0.0179633, "Field Reading"=-1.3894e-07}, {-0.0199615, "Field Reading"=-1.5446e-07}, {-0.0219611, "Field Reading"=-1.70002e-07}, {-0.0239586, "Field Reading"=-1.85629e-07}, {-0.0259606, "Field Reading"=-2.01277e-07}, {-0.0279626, "Field Reading"=-2.16959e-07}, {-0.0299578, "Field Reading"=-2.32681e-07}, {-0.031959, "Field Reading"=-2.48447e-07}, {-0.0339592, "Field Reading"=-2.64261e-07}, {-0.0359603, "Field Reading"=-2.80151e-07}, {-0.0379647, "Field Reading"=-2.9609e-07}, {-0.0399635, "Field Reading"=-3.12036e-07}, {-0.0419601, "Field Reading"=-3.2803e-07}, {-0.0439643, "Field Reading"=-3.44121e-07}, {-0.0459585, "Field Reading"=-3.60293e-07}, {-0.0479606, "Field Reading"=-3.76556e-07}, {-0.0499626, "Field Reading"=-3.92795e-07}, {-0.0519609, "Field Reading"=-4.09108e-07}, {-0.0539638, "Field Reading"=-4.25564e-07}, {-0.0559645, "Field Reading"=-4.41993e-07}, {-0.0579646, "Field Reading"=-4.58556e-07}, {-0.0599606, "Field Reading"=-4.75131e-07}, {-0.0619605, "Field Reading"=-4.91767e-07}, {-0.0639597, "Field Reading"=-5.08547e-07}, {-0.0659617, "Field Reading"=-5.25382e-07}, {-0.06796, "Field Reading"=-5.42193e-07}, {-0.0699609, "Field Reading"=-5.59162e-07}, {-0.0719576, "Field Reading"=-5.76215e-07}, {-0.0739591, "Field Reading"=-5.93372e-07}, {-0.0759554, "Field Reading"=-6.10523e-07}, {-0.0779573, "Field Reading"=-6.27763e-07}, {-0.0799575, "Field Reading"=-6.45252e-07}, {-0.0819596, "Field Reading"=-6.62657e-07}, {-0.0839633, "Field Reading"=-6.80222e-07}, {-0.0859642, "Field Reading"=-6.97947e-07}, {-0.0879685, "Field Reading"=-7.15707e-07}, {-0.0899625, "Field Reading"=-7.33331e-07}, {-0.091961, "Field Reading"=-7.51292e-07}, {-0.0939611, "Field Reading"=-7.69095e-07}, {-0.0959609, "Field Reading"=-7.87462e-07}, {-0.097957, "Field Reading"=-8.05664e-07}, {-0.0999584, "Field Reading"=-8.23921e-07}, {-0.101958, "Field Reading"=-8.42313e-07}, {-0.10396, "Field Reading"=-8.60184e-07}, {-0.105956, "Field Reading"=-8.78728e-07}, {-0.107955, "Field Reading"=-8.98077e-07}, {-0.109957, "Field Reading"=-9.16917e-07}, {-0.111957, "Field Reading"=-9.35788e-07}, {-0.113957, "Field Reading"=-9.54994e-07}, {-0.115961, "Field Reading"=-9.7397e-07}, {-0.117958, "Field Reading"=-9.93295e-07}, {-0.119958, "Field Reading"=-1.01251e-06}, {-0.121958, "Field Reading"=-1.03197e-06}, {-0.123962, "Field Reading"=-1.05169e-06}, {-0.12596, "Field Reading"=-1.07141e-06}, {-0.127961, "Field Reading"=-1.0911e-06}, {-0.129961, "Field Reading"=-1.11108e-06}, {-0.131962, "Field Reading"=-1.13132e-06}, {-0.133958, "Field Reading"=-1.15127e-06}, {-0.135959, "Field Reading"=-1.1715e-06}, {-0.137961, "Field Reading"=-1.19203e-06}, {-0.139958, "Field Reading"=-1.21255e-06}, {-0.141961, "Field Reading"=-1.23343e-06}, {-0.143963, "Field Reading"=-1.25429e-06}, {-0.145961, "Field Reading"=-1.27517e-06}, {-0.147961, "Field Reading"=-1.29628e-06}, {-0.14996, "Field Reading"=-1.3175e-06}, {-0.151959, "Field Reading"=-1.33889e-06}, {-0.15396, "Field Reading"=-1.36038e-06}, {-0.155959, "Field Reading"=-1.38212e-06}, {-0.15796, "Field Reading"=-1.40375e-06}, {-0.15996, "Field Reading"=-1.42566e-06}, {-0.161958, "Field Reading"=-1.44773e-06}, {-0.163955, "Field Reading"=-1.4698e-06}, {-0.165959, "Field Reading"=-1.49253e-06}, {-0.167959, "Field Reading"=-1.51493e-06}, {-0.16996, "Field Reading"=-1.53748e-06}, {-0.171962, "Field Reading"=-1.56064e-06}, {-0.173959, "Field Reading"=-1.58369e-06}, {-0.17596, "Field Reading"=-1.60676e-06}, {-0.177961, "Field Reading"=-1.63014e-06}, {-0.179957, "Field Reading"=-1.65404e-06}, {-0.181956, "Field Reading"=-1.67748e-06}, {-0.183955, "Field Reading"=-1.70078e-06}, {-0.185953, "Field Reading"=-1.72532e-06}, {-0.187954, "Field Reading"=-1.74944e-06}, {-0.189952, "Field Reading"=-1.77354e-06}, {-0.191953, "Field Reading"=-1.79739e-06}, {-0.193951, "Field Reading"=-1.82278e-06}, {-0.195952, "Field Reading"=-1.84792e-06}, {-0.197953, "Field Reading"=-1.87288e-06}, {-0.199955, "Field Reading"=-1.89798e-06}, {-0.20198, "Field Reading"=-1.92387e-06}, {-0.203947, "Field Reading"=-1.94924e-06}, {-0.205948, "Field Reading"=-1.97524e-06}, {-0.207951, "Field Reading"=-2.0016e-06}, {-0.209952, "Field Reading"=-2.02721e-06}, {-0.211962, "Field Reading"=-2.05438e-06}, {-0.213962, "Field Reading"=-2.08069e-06}, {-0.215967, "Field Reading"=-2.10812e-06}, {-0.217971, "Field Reading"=-2.13484e-06}, {-0.219975, "Field Reading"=-2.16222e-06}, {-0.221975, "Field Reading"=-2.18924e-06}, {-0.223982, "Field Reading"=-2.21791e-06}, {-0.22595, "Field Reading"=-2.24532e-06}, {-0.22795, "Field Reading"=-2.27423e-06}, {-0.229955, "Field Reading"=-2.30218e-06}, {-0.231961, "Field Reading"=-2.33101e-06}, {-0.233959, "Field Reading"=-2.36033e-06}, {-0.235963, "Field Reading"=-2.38897e-06}, {-0.237971, "Field Reading"=-2.41818e-06}, {-0.239972, "Field Reading"=-2.44859e-06}, {-0.241978, "Field Reading"=-2.47812e-06}, {-0.24398, "Field Reading"=-2.5085e-06}, {-0.245986, "Field Reading"=-2.53899e-06}, {-0.247953, "Field Reading"=-2.56917e-06}, {-0.249964, "Field Reading"=-2.60054e-06}, {-0.251966, "Field Reading"=-2.632e-06}, {-0.253968, "Field Reading"=-2.66285e-06}, {-0.255967, "Field Reading"=-2.69506e-06}, {-0.257976, "Field Reading"=-2.72725e-06}, {-0.259975, "Field Reading"=-2.75922e-06}, {-0.261979, "Field Reading"=-2.79206e-06}, {-0.26398, "Field Reading"=-2.8244e-06}, {-0.265988, "Field Reading"=-2.8583e-06}, {-0.267989, "Field Reading"=-2.89226e-06}, {-0.269958, "Field Reading"=-2.92528e-06}, {-0.27196, "Field Reading"=-2.95905e-06}, {-0.273967, "Field Reading"=-2.99385e-06}, {-0.27597, "Field Reading"=-3.02935e-06}, {-0.277973, "Field Reading"=-3.06401e-06}, {-0.279978, "Field Reading"=-3.09926e-06}, {-0.28198, "Field Reading"=-3.13502e-06}, {-0.283984, "Field Reading"=-3.17102e-06}, {-0.285989, "Field Reading"=-3.20754e-06}, {-0.287992, "Field Reading"=-3.24408e-06}, {-0.289996, "Field Reading"=-3.28065e-06}, {-0.291996, "Field Reading"=-3.31901e-06}, {-0.293969, "Field Reading"=-3.35612e-06}, {-0.29597, "Field Reading"=-3.3943e-06}, {-0.297976, "Field Reading"=-3.43278e-06}, {-0.299977, "Field Reading"=-3.47195e-06}, {-0.301984, "Field Reading"=-3.51104e-06}, {-0.303985, "Field Reading"=-3.55078e-06}, {-0.305994, "Field Reading"=-3.59065e-06}, {-0.307994, "Field Reading"=-3.63137e-06}, {-0.309994, "Field Reading"=-3.67132e-06}, {-0.312002, "Field Reading"=-3.71336e-06}, {-0.314005, "Field Reading"=-3.75496e-06}, {-0.31597, "Field Reading"=-3.79568e-06}, {-0.317976, "Field Reading"=-3.83916e-06}, {-0.319977, "Field Reading"=-3.88239e-06}, {-0.321985, "Field Reading"=-3.92522e-06}, {-0.323984, "Field Reading"=-3.96845e-06}, {-0.325988, "Field Reading"=-4.01356e-06}, {-0.327989, "Field Reading"=-4.05738e-06}, {-0.329999, "Field Reading"=-4.1023e-06}, {-0.332, "Field Reading"=-4.14897e-06}, {-0.33401, "Field Reading"=-4.19475e-06}, {-0.336008, "Field Reading"=-4.24067e-06}, {-0.337976, "Field Reading"=-4.28718e-06}, {-0.339982, "Field Reading"=-4.33432e-06}, {-0.341988, "Field Reading"=-4.38359e-06}, {-0.343988, "Field Reading"=-4.43085e-06}, {-0.345992, "Field Reading"=-4.47957e-06}, {-0.348, "Field Reading"=-4.52856e-06}, {-0.350002, "Field Reading"=-4.57877e-06}, {-0.352004, "Field Reading"=-4.63038e-06}, {-0.354007, "Field Reading"=-4.68012e-06}, {-0.356012, "Field Reading"=-4.73153e-06}, {-0.358017, "Field Reading"=-4.78425e-06}, {-0.359986, "Field Reading"=-4.83528e-06}, {-0.361982, "Field Reading"=-4.88795e-06}, {-0.363986, "Field Reading"=-4.9417e-06}, {-0.365991, "Field Reading"=-4.99666e-06}, {-0.367996, "Field Reading"=-5.05079e-06}, {-0.369992, "Field Reading"=-5.10587e-06}, {-0.371998, "Field Reading"=-5.16207e-06}, {-0.373996, "Field Reading"=-5.21788e-06}, {-0.376007, "Field Reading"=-5.27575e-06}, {-0.378006, "Field Reading"=-5.33245e-06}, {-0.380014, "Field Reading"=-5.39207e-06}, {-0.382015, "Field Reading"=-5.4495e-06}, {-0.383981, "Field Reading"=-5.51006e-06}, {-0.385979, "Field Reading"=-5.56854e-06}, {-0.387997, "Field Reading"=-5.62959e-06}, {-0.389992, "Field Reading"=-5.69228e-06}, {-0.392002, "Field Reading"=-5.7535e-06}, {-0.394008, "Field Reading"=-5.81608e-06}, {-0.396009, "Field Reading"=-5.87874e-06}, {-0.398009, "Field Reading"=-5.94343e-06}, {-0.40002, "Field Reading"=-6.00767e-06}, {-0.40202, "Field Reading"=-6.07371e-06}, {-0.404029, "Field Reading"=-6.13994e-06}, {-0.405987, "Field Reading"=-6.2049e-06}, {-0.407992, "Field Reading"=-6.2724e-06}, {-0.409994, "Field Reading"=-6.3413e-06}, {-0.412001, "Field Reading"=-6.41059e-06}, {-0.414003, "Field Reading"=-6.4799e-06}, {-0.41601, "Field Reading"=-6.55082e-06}, {-0.418015, "Field Reading"=-6.62283e-06}, {-0.420025, "Field Reading"=-6.69402e-06}, {-0.422024, "Field Reading"=-6.76639e-06}, {-0.424028, "Field Reading"=-6.83923e-06}, {-0.426028, "Field Reading"=-6.91296e-06}, {-0.427994, "Field Reading"=-6.98807e-06}, {-0.430001, "Field Reading"=-7.06307e-06}, {-0.432007, "Field Reading"=-7.13871e-06}, {-0.434006, "Field Reading"=-7.21755e-06}, {-0.436012, "Field Reading"=-7.2966e-06}, {-0.438009, "Field Reading"=-7.37517e-06}, {-0.440016, "Field Reading"=-7.45462e-06}, {-0.442016, "Field Reading"=-7.53522e-06}, {-0.444021, "Field Reading"=-7.61865e-06}, {-0.446023, "Field Reading"=-7.69813e-06}, {-0.44803, "Field Reading"=-7.78155e-06}, {-0.449998, "Field Reading"=-7.86404e-06}, {-0.452002, "Field Reading"=-7.94988e-06}, {-0.454003, "Field Reading"=-8.03416e-06}, {-0.456008, "Field Reading"=-8.12164e-06}, {-0.458016, "Field Reading"=-8.2097e-06}, {-0.460012, "Field Reading"=-8.2986e-06}, {-0.462015, "Field Reading"=-8.38658e-06}, {-0.464016, "Field Reading"=-8.47619e-06}, {-0.466018, "Field Reading"=-8.56746e-06}, {-0.468027, "Field Reading"=-8.66097e-06}, {-0.470028, "Field Reading"=-8.75657e-06}, {-0.471994, "Field Reading"=-8.84793e-06}, {-0.473999, "Field Reading"=-8.94409e-06}, {-0.476006, "Field Reading"=-9.03661e-06}, {-0.478008, "Field Reading"=-9.13507e-06}, {-0.480011, "Field Reading"=-9.2336e-06}, {-0.482016, "Field Reading"=-9.33118e-06}, {-0.484016, "Field Reading"=-9.43108e-06}, {-0.486025, "Field Reading"=-9.53591e-06}, {-0.488023, "Field Reading"=-9.63746e-06}, {-0.490024, "Field Reading"=-9.73938e-06}, {-0.492028, "Field Reading"=-9.84415e-06}, {-0.494033, "Field Reading"=-9.95089e-06}, {-0.496014, "Field Reading"=-1.00548e-05}, {-0.498009, "Field Reading"=-1.016e-05}, {-0.500013, "Field Reading"=-1.02672e-05}, {-0.498004, "Field Reading"=-1.0158e-05}, {-0.496006, "Field Reading"=-1.00512e-05}, {-0.49403, "Field Reading"=-9.94588e-06}, {-0.492022, "Field Reading"=-9.83877e-06}, {-0.490024, "Field Reading"=-9.73414e-06}, {-0.488019, "Field Reading"=-9.62893e-06}, {-0.486018, "Field Reading"=-9.52456e-06}, {-0.484006, "Field Reading"=-9.42148e-06}, {-0.48201, "Field Reading"=-9.32139e-06}, {-0.480006, "Field Reading"=-9.22255e-06}, {-0.478006, "Field Reading"=-9.12336e-06}, {-0.475996, "Field Reading"=-9.02526e-06}, {-0.473993, "Field Reading"=-8.9275e-06}, {-0.47199, "Field Reading"=-8.83159e-06}, {-0.470021, "Field Reading"=-8.73904e-06}, {-0.468024, "Field Reading"=-8.64506e-06}, {-0.466013, "Field Reading"=-8.55196e-06}, {-0.464014, "Field Reading"=-8.45992e-06}, {-0.462008, "Field Reading"=-8.36928e-06}, {-0.460009, "Field Reading"=-8.27766e-06}, {-0.458008, "Field Reading"=-8.19078e-06}, {-0.456002, "Field Reading"=-8.10396e-06}, {-0.453998, "Field Reading"=-8.01848e-06}, {-0.451999, "Field Reading"=-7.93287e-06}, {-0.449997, "Field Reading"=-7.84528e-06}, {-0.448026, "Field Reading"=-7.76347e-06}, {-0.446018, "Field Reading"=-7.67925e-06}, {-0.444018, "Field Reading"=-7.59732e-06}, {-0.442013, "Field Reading"=-7.51619e-06}, {-0.440015, "Field Reading"=-7.43505e-06}, {-0.438011, "Field Reading"=-7.35462e-06}, {-0.436011, "Field Reading"=-7.2752e-06}, {-0.434004, "Field Reading"=-7.19745e-06}, {-0.432005, "Field Reading"=-7.11976e-06}, {-0.429998, "Field Reading"=-7.0442e-06}, {-0.427987, "Field Reading"=-6.9683e-06}, {-0.426018, "Field Reading"=-6.89316e-06}, {-0.424016, "Field Reading"=-6.8208e-06}, {-0.422013, "Field Reading"=-6.74692e-06}, {-0.420016, "Field Reading"=-6.67309e-06}, {-0.41801, "Field Reading"=-6.60241e-06}, {-0.416011, "Field Reading"=-6.53093e-06}, {-0.414001, "Field Reading"=-6.46126e-06}, {-0.412005, "Field Reading"=-6.39071e-06}, {-0.409998, "Field Reading"=-6.32311e-06}, {-0.407997, "Field Reading"=-6.25308e-06}, {-0.405994, "Field Reading"=-6.18582e-06}, {-0.404031, "Field Reading"=-6.11979e-06}, {-0.402021, "Field Reading"=-6.05325e-06}, {-0.400021, "Field Reading"=-5.98713e-06}, {-0.398012, "Field Reading"=-5.92442e-06}, {-0.396014, "Field Reading"=-5.86035e-06}, {-0.394009, "Field Reading"=-5.79865e-06}, {-0.391997, "Field Reading"=-5.73573e-06}, {-0.389995, "Field Reading"=-5.67408e-06}, {-0.387993, "Field Reading"=-5.61271e-06}, {-0.386003, "Field Reading"=-5.55213e-06}, {-0.38398, "Field Reading"=-5.49147e-06}, {-0.382012, "Field Reading"=-5.43224e-06}, {-0.380008, "Field Reading"=-5.37231e-06}, {-0.37801, "Field Reading"=-5.3149e-06}, {-0.376007, "Field Reading"=-5.25613e-06}, {-0.373993, "Field Reading"=-5.19815e-06}, {-0.371995, "Field Reading"=-5.14277e-06}, {-0.369989, "Field Reading"=-5.08762e-06}, {-0.367993, "Field Reading"=-5.0324e-06}, {-0.365987, "Field Reading"=-4.97652e-06}, {-0.36398, "Field Reading"=-4.92245e-06}, {-0.361978, "Field Reading"=-4.86939e-06}, {-0.359975, "Field Reading"=-4.81625e-06}, {-0.358009, "Field Reading"=-4.76554e-06}, {-0.356007, "Field Reading"=-4.71395e-06}, {-0.354001, "Field Reading"=-4.66217e-06}, {-0.352004, "Field Reading"=-4.61015e-06}, {-0.349996, "Field Reading"=-4.56099e-06}, {-0.347993, "Field Reading"=-4.51113e-06}, {-0.345985, "Field Reading"=-4.46272e-06}, {-0.343982, "Field Reading"=-4.41389e-06}, {-0.341982, "Field Reading"=-4.36575e-06}, {-0.339976, "Field Reading"=-4.31822e-06}, {-0.337977, "Field Reading"=-4.27138e-06}, {-0.336009, "Field Reading"=-4.22493e-06}, {-0.334004, "Field Reading"=-4.17858e-06}, {-0.332005, "Field Reading"=-4.13269e-06}, {-0.330001, "Field Reading"=-4.08723e-06}, {-0.327996, "Field Reading"=-4.04084e-06}, {-0.326, "Field Reading"=-3.99852e-06}, {-0.323995, "Field Reading"=-3.95354e-06}, {-0.321995, "Field Reading"=-3.91047e-06}, {-0.319988, "Field Reading"=-3.86675e-06}, {-0.317987, "Field Reading"=-3.82483e-06}, {-0.315977, "Field Reading"=-3.78259e-06}, {-0.314014, "Field Reading"=-3.74195e-06}, {-0.31201, "Field Reading"=-3.70048e-06}, {-0.310004, "Field Reading"=-3.65905e-06}, {-0.308003, "Field Reading"=-3.61745e-06}, {-0.306002, "Field Reading"=-3.57704e-06}, {-0.304001, "Field Reading"=-3.53731e-06}, {-0.301998, "Field Reading"=-3.49808e-06}, {-0.299986, "Field Reading"=-3.45918e-06}, {-0.297984, "Field Reading"=-3.42014e-06}, {-0.295979, "Field Reading"=-3.38109e-06}, {-0.293978, "Field Reading"=-3.34336e-06}, {-0.29201, "Field Reading"=-3.30672e-06}, {-0.290004, "Field Reading"=-3.26907e-06}, {-0.288002, "Field Reading"=-3.23205e-06}, {-0.285999, "Field Reading"=-3.19511e-06}, {-0.283993, "Field Reading"=-3.15903e-06}, {-0.281991, "Field Reading"=-3.12288e-06}, {-0.279981, "Field Reading"=-3.08763e-06}, {-0.27798, "Field Reading"=-3.05131e-06}, {-0.275977, "Field Reading"=-3.01746e-06}, {-0.273973, "Field Reading"=-2.9825e-06}, {-0.271975, "Field Reading"=-2.94858e-06}, {-0.269975, "Field Reading"=-2.91443e-06}, {-0.268002, "Field Reading"=-2.8813e-06}, {-0.266006, "Field Reading"=-2.84761e-06}, {-0.263996, "Field Reading"=-2.81311e-06}, {-0.261996, "Field Reading"=-2.7818e-06}, {-0.259994, "Field Reading"=-2.74926e-06}, {-0.25799, "Field Reading"=-2.71728e-06}, {-0.255981, "Field Reading"=-2.68503e-06}, {-0.253979, "Field Reading"=-2.65345e-06}, {-0.251976, "Field Reading"=-2.62202e-06}, {-0.249978, "Field Reading"=-2.59053e-06}, {-0.247975, "Field Reading"=-2.55993e-06}, {-0.245998, "Field Reading"=-2.52988e-06}, {-0.243995, "Field Reading"=-2.49943e-06}, {-0.241994, "Field Reading"=-2.46884e-06}, {-0.239988, "Field Reading"=-2.43967e-06}, {-0.237987, "Field Reading"=-2.40946e-06}, {-0.235979, "Field Reading"=-2.38021e-06}, {-0.23398, "Field Reading"=-2.35131e-06}, {-0.231977, "Field Reading"=-2.32246e-06}, {-0.229973, "Field Reading"=-2.29412e-06}, {-0.227966, "Field Reading"=-2.26498e-06}, {-0.225965, "Field Reading"=-2.23731e-06}, {-0.224, "Field Reading"=-2.20817e-06}, {-0.221994, "Field Reading"=-2.1823e-06}, {-0.219993, "Field Reading"=-2.15469e-06}, {-0.217984, "Field Reading"=-2.12749e-06}, {-0.215986, "Field Reading"=-2.10025e-06}, {-0.213981, "Field Reading"=-2.074e-06}, {-0.21198, "Field Reading"=-2.04703e-06}, {-0.20997, "Field Reading"=-2.02085e-06}, {-0.207967, "Field Reading"=-1.99409e-06}, {-0.205961, "Field Reading"=-1.96656e-06}, {-0.20396, "Field Reading"=-1.94106e-06}, {-0.20199, "Field Reading"=-1.91734e-06}, {-0.199959, "Field Reading"=-1.89118e-06}, {-0.19796, "Field Reading"=-1.86606e-06}, {-0.195959, "Field Reading"=-1.84121e-06}, {-0.193956, "Field Reading"=-1.81656e-06}, {-0.191961, "Field Reading"=-1.79207e-06}, {-0.18996, "Field Reading"=-1.76738e-06}, {-0.187961, "Field Reading"=-1.74271e-06}, {-0.185959, "Field Reading"=-1.71906e-06}, {-0.183961, "Field Reading"=-1.69483e-06}, {-0.181961, "Field Reading"=-1.67114e-06}, {-0.179962, "Field Reading"=-1.64739e-06}, {-0.177968, "Field Reading"=-1.62414e-06}, {-0.175967, "Field Reading"=-1.60091e-06}, {-0.173965, "Field Reading"=-1.57795e-06}, {-0.171965, "Field Reading"=-1.55495e-06}, {-0.169964, "Field Reading"=-1.53219e-06}, {-0.167962, "Field Reading"=-1.50961e-06}, {-0.165963, "Field Reading"=-1.48677e-06}, {-0.163964, "Field Reading"=-1.4645e-06}, {-0.161966, "Field Reading"=-1.44272e-06}, {-0.159966, "Field Reading"=-1.42032e-06}, {-0.157964, "Field Reading"=-1.39883e-06}, {-0.155961, "Field Reading"=-1.37707e-06}, {-0.15396, "Field Reading"=-1.35544e-06}, {-0.151961, "Field Reading"=-1.33422e-06}, {-0.149963, "Field Reading"=-1.3129e-06}, {-0.147966, "Field Reading"=-1.29178e-06}, {-0.145965, "Field Reading"=-1.26965e-06}, {-0.143965, "Field Reading"=-1.2487e-06}, {-0.141965, "Field Reading"=-1.22805e-06}, {-0.139967, "Field Reading"=-1.20731e-06}, {-0.137966, "Field Reading"=-1.18784e-06}, {-0.135962, "Field Reading"=-1.16738e-06}, {-0.133963, "Field Reading"=-1.14734e-06}, {-0.131967, "Field Reading"=-1.12702e-06}, {-0.129969, "Field Reading"=-1.10701e-06}, {-0.127968, "Field Reading"=-1.08721e-06}, {-0.125967, "Field Reading"=-1.06743e-06}, {-0.123964, "Field Reading"=-1.04776e-06}, {-0.121962, "Field Reading"=-1.02808e-06}, {-0.119961, "Field Reading"=-1.00877e-06}, {-0.117965, "Field Reading"=-9.89525e-07}, {-0.115963, "Field Reading"=-9.70315e-07}, {-0.113966, "Field Reading"=-9.51298e-07}, {-0.111967, "Field Reading"=-9.32167e-07}, {-0.109966, "Field Reading"=-9.13391e-07}, {-0.107968, "Field Reading"=-8.94734e-07}, {-0.105968, "Field Reading"=-8.7613e-07}, {-0.103971, "Field Reading"=-8.5756e-07}, {-0.101971, "Field Reading"=-8.39123e-07}, {-0.0999734, "Field Reading"=-8.20844e-07}, {-0.0979708, "Field Reading"=-8.02632e-07}, {-0.0959695, "Field Reading"=-7.84451e-07}, {-0.0939698, "Field Reading"=-7.65984e-07}, {-0.0919739, "Field Reading"=-7.48479e-07}, {-0.0899753, "Field Reading"=-7.3067e-07}, {-0.0879776, "Field Reading"=-7.12968e-07}, {-0.0859743, "Field Reading"=-6.95278e-07}, {-0.0839735, "Field Reading"=-6.77688e-07}, {-0.0819712, "Field Reading"=-6.60198e-07}, {-0.0799742, "Field Reading"=-6.42864e-07}, {-0.0779748, "Field Reading"=-6.25532e-07}, {-0.0759753, "Field Reading"=-6.08285e-07}, {-0.0739803, "Field Reading"=-5.9111e-07}, {-0.0719775, "Field Reading"=-5.74021e-07}, {-0.0699769, "Field Reading"=-5.57066e-07}, {-0.067973, "Field Reading"=-5.40169e-07}, {-0.0659737, "Field Reading"=-5.23334e-07}, {-0.0639725, "Field Reading"=-5.06528e-07}, {-0.0619723, "Field Reading"=-4.89931e-07}, {-0.0599715, "Field Reading"=-4.73307e-07}, {-0.0579734, "Field Reading"=-4.56786e-07}, {-0.0559742, "Field Reading"=-4.40366e-07}, {-0.0539768, "Field Reading"=-4.2397e-07}, {-0.0519753, "Field Reading"=-4.07661e-07}, {-0.0499765, "Field Reading"=-3.91372e-07}, {-0.0479753, "Field Reading"=-3.75143e-07}, {-0.0459754, "Field Reading"=-3.58982e-07}, {-0.0439772, "Field Reading"=-3.42918e-07}, {-0.0419794, "Field Reading"=-3.26899e-07}, {-0.0399775, "Field Reading"=-3.10925e-07}, {-0.0379795, "Field Reading"=-2.95012e-07}, {-0.0359774, "Field Reading"=-2.79135e-07}, {-0.0339733, "Field Reading"=-2.63266e-07}, {-0.0319713, "Field Reading"=-2.47447e-07}, {-0.0299684, "Field Reading"=-2.31705e-07}, {-0.0279702, "Field Reading"=-2.1602e-07}, {-0.0259681, "Field Reading"=-2.00371e-07}, {-0.0239672, "Field Reading"=-1.84745e-07}, {-0.0219603, "Field Reading"=-1.69154e-07}, {-0.0199614, "Field Reading"=-1.53613e-07}, {-0.0179615, "Field Reading"=-1.38108e-07}, {-0.0159585, "Field Reading"=-1.22626e-07}, {-0.0139637, "Field Reading"=-1.07239e-07}, {-0.0119623, "Field Reading"=-9.18377e-08}, {-0.00996189, "Field Reading"=-7.6484e-08}, {-0.00796263, "Field Reading"=-6.11066e-08}, {-0.00595863, "Field Reading"=-4.57565e-08}, {-0.00395613, "Field Reading"=-3.04287e-08}, {-0.00195336, "Field Reading"=-1.51156e-08}]
  out "data":dbl[](array[numeric])=[-0.00195336, -1.51156e-08, 129228.0822461563]
  in  "Source meter K2636B":refnum<visa-resource-name>="GPIB0::26::INSTR"
  in  "Step":dbl[](array[numeric])=[0.002, 0.002, 0.002] min=-3000.0 max=3000.0 format="%.1e"
  in  "To":dbl[](array[numeric])=[0.5, -0.5, 0.0] min=-3000.0 max=3000.0 format="%.1e"
  in  "From":dbl[](array[numeric])=[0.0, 0.5, -0.5] min=-3000.0 max=3000.0 format="%.1e"
  in  "file name":string="007_MA1981_Dev007_V(I)_300K"
  out "File path":path=path "D:/Pranava/Data/STS/MA1981/006_MA1981_Dev006_V(I)_300K.dat"
  # ".dat"
  # "2-point sense"
  # "Set Voltage (V)"
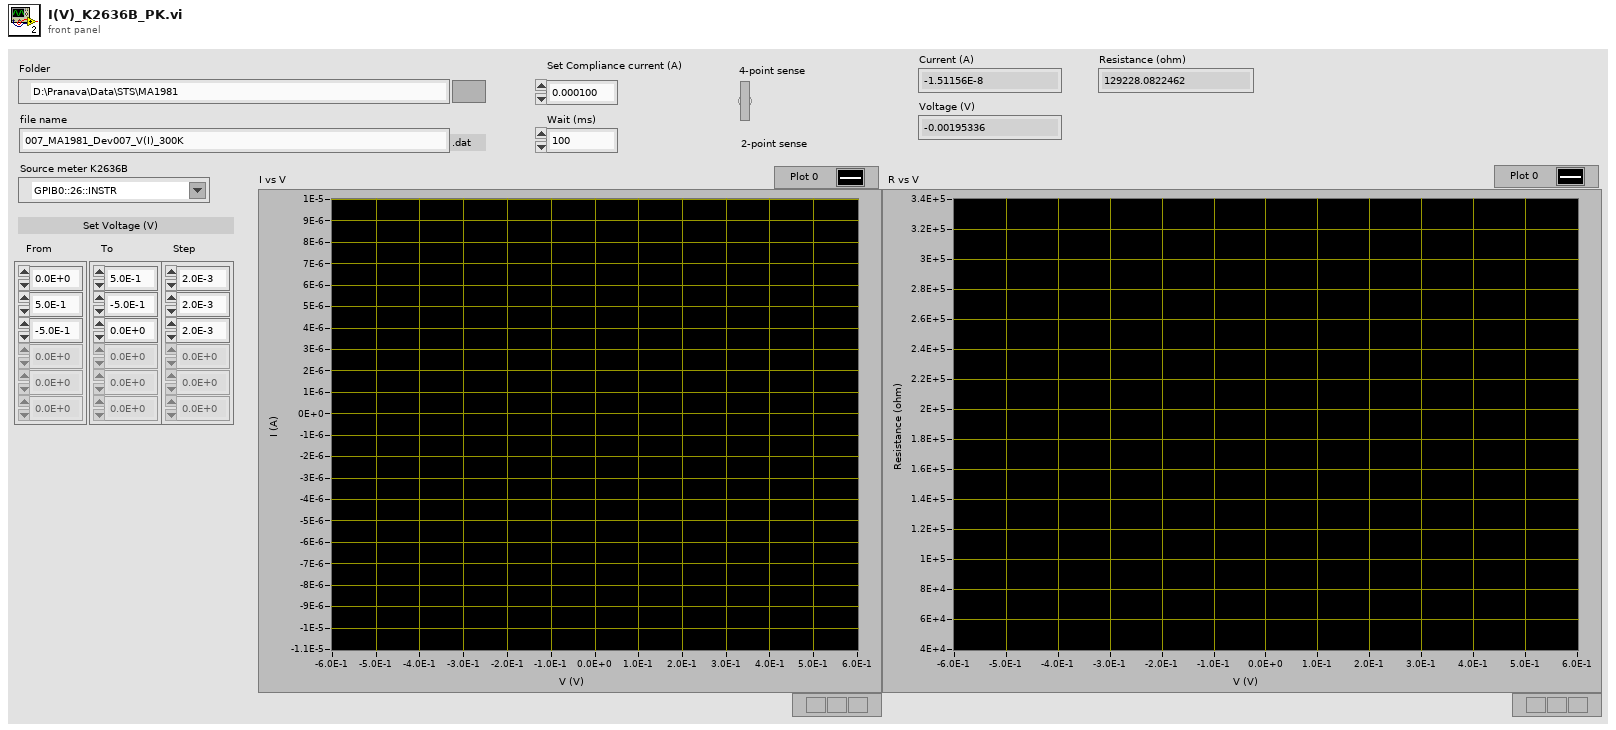
[diagram p1: front panel]
types:
  T1 = enum16{"open", "replace", "create", "open or create", "replace or create", "replace or create with confirmation"}
  T2 = cluster{"Last Voltage (V)":dbl, "Last Current (A)":dbl}
  T3 = cluster{"Last Voltage (V)":dbl, "Last Current (A)":dbl}[]
  T4 = cluster{"Last Voltage (V)":dbl, "Field Reading":dbl}[]
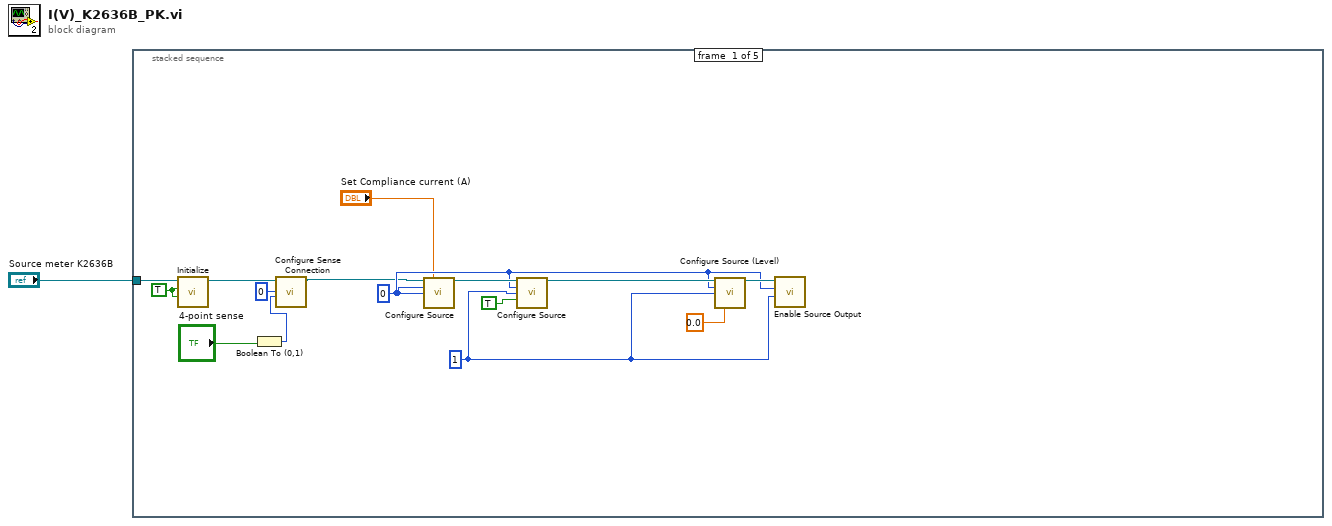
[diagram p0: block diagram]
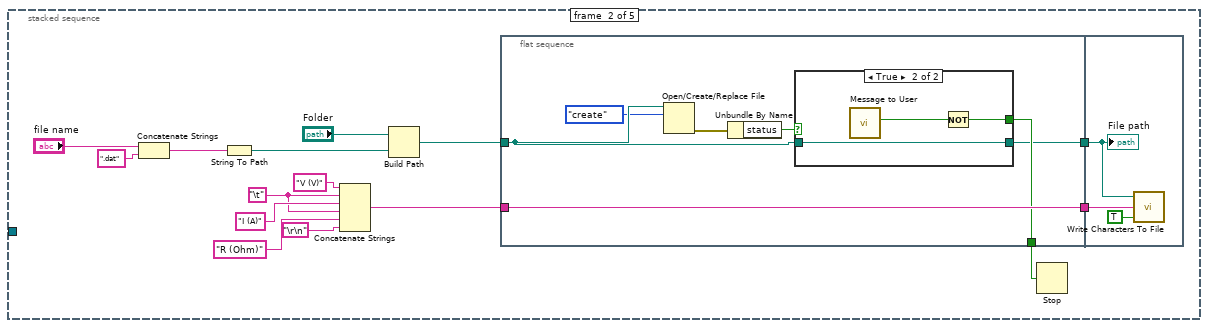
[diagram p2: hidden frame]
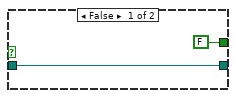
[diagram p3: hidden frame]
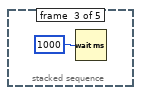
[diagram p4: hidden frame]
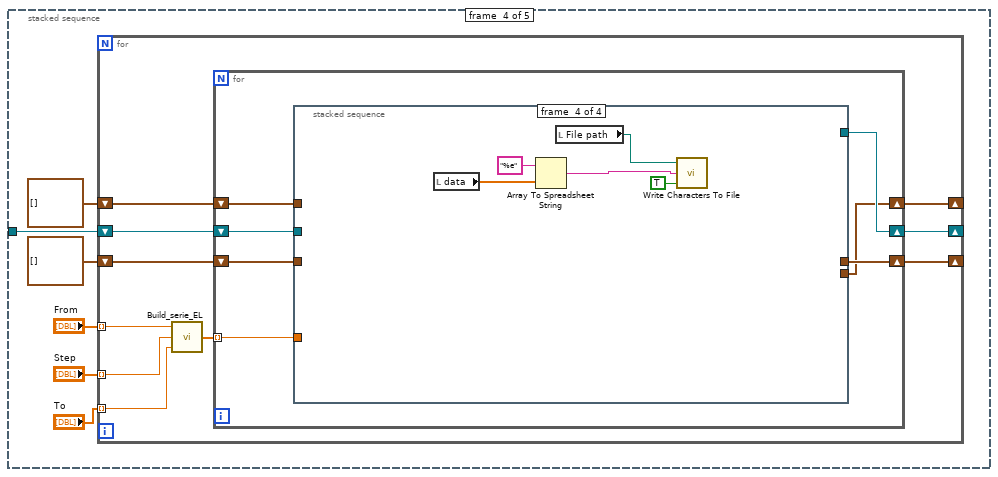
[diagram p5: hidden frame]
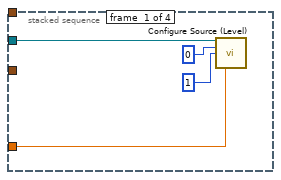
[diagram p6: hidden frame]
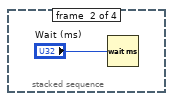
[diagram p7: hidden frame]
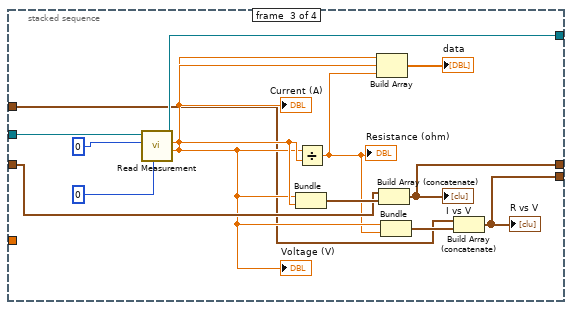
[diagram p8: hidden frame]
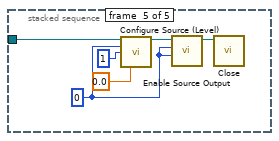
[diagram p9: hidden frame]
diagram:
  n1 = stacked-sequence {
    tunnel: "Source meter K2636B" -> [w16 _ _ w50 w98]
    frame #0 {
      w8 = TRUE
      w11 = 0
      w9 = 1
      n2 = call <instrlib>:"Initialize.vi"("Reset (True)"=w8, "ID Query (True)"=w8, "VISA resource name"=w16) -> ("VISA resource name out"=w6:refnum<visa-resource-name>)  [unwired: 7 in, 1 out]
      n3 = Boolean To (0,1)(Boolean="4-point sense") -> (0, 1=w2:i16)
      n4 = call <instrlib>:"Configure Sense Connection.vi"("Sense Mode (0: Local Sense)"=w2, "Source Measure Unit Channel (0: Channel A)"=0, "VISA resource name"=w6) -> ("VISA resource name out"=w5:refnum<visa-resource-name>)  [unwired: 7 in, 1 out]
      n5 = call-poly <instrlib>:"Configure Source.vi"("VISA resource name"=w5, "Current Limit (0.1 A)"="Set Compliance current (A)", "Source Measure Unit Channel (0: Channel A)"=w11, "Limit Type (1: Voltage)"=w11) -> ("VISA resource name out"=w15:refnum<visa-resource-name>)  [unwired: 10 in, 1 out]
      n6 = call-poly <instrlib>:"Configure Source.vi"("VISA resource name"=w15, "Source Measure Unit Channel (0: Channel A)"=w11, "Range Type (1: Voltage)"=w9, "Auto Range (T: Enable)"=TRUE) -> ("VISA resource name out"=w14:refnum<visa-resource-name>)  [unwired: 10 in, 1 out]
      n7 = call <instrlib>:"Configure Source (Level).vi"("VISA resource name"=w14, "Source Measure Unit Channel (0: Channel A)"=w11, "Level Type (1: Voltage)"=w9, "Voltage Level (0 V)"=0.0) -> ("VISA resource name out"=w13:refnum<visa-resource-name>)  [unwired: 10 in, 1 out]
      n8 = call <instrlib>:"Enable Source Output.vi"("Output Mode (0: Turn off)"=w9, "Source Measure Unit Channel (0: Channel A)"=w11, "VISA resource name"=w13) -> ()  [unwired: 7 in, 2 out]
    }
    frame #1 {
      w22 = "\t"
      n9 = Concatenate Strings("file name", ".dat" ("string")) -> (w28:string)
      n10 = String To Path(string=w28) -> (path=w18:path)
      n11 = Concatenate Strings("V (V)" ("string"), w22, "I (A)" ("string"), w22, "R (Ohm)" ("string"), "\r\n") -> (w29:string)
      n12 = Build Path(base path="Folder", name or relative path=w18) -> (appended path=w17:path)
      n13 = flat-sequence {
        tunnel: w17 -> [w35]
        tunnel: w29 -> [w38]
        tunnel: [w38] -> w31
        tunnel: [w37] -> w26
        tunnel: [w36] -> w30
        tunnel: w31 -> [w45]
        tunnel: w30 -> [w44]
        frame #0 {
          n14 = Open/Create/Replace File(file path (use dialog)=w35, operation (0:open)=T1."create") -> (error out=w34:errorcluster)  [unwired: 4 in, 2 out]
          n15 = Unbundle By Name(w34) -> ("status"=w32:bool)
          n16 = case shown="True" w32 {
            tunnel: [FALSE ("Yes") w42] -> w37
            tunnel: [w39 w41] -> w36
            tunnel: w35 -> [w39 w41]
            frame False {
            }
            frame True {
              n17 = call "Message to User"() -> ("Yes"=w43:bool)  [unwired: 10 in, 1 out]
              n18 = Not(x=w43) -> (.not. x?=w42:bool)
            }
          }
        }
        frame #1 {
          n19 = call <vilib>:"Write Characters To File.vi"("append to file? (new file:F)"=TRUE, "character string"=w45, "file path (dialog if empty)"=w44) -> ()  [unwired: 2 in, 1 out]
          "File path" <- w44
        }
      }
      n20 = Stop(stop? (T)=w26) -> ()
    }
    frame #2 {
      n21 = Wait (ms)(milliseconds to wait=u32 1000) -> ()  [unwired: 1 out]
    }
    frame #3 {
      n22 = for {
        tunnel: "From" -> [w59] mode=indexing
        tunnel: "To" -> [w58] mode=indexing
        tunnel: "Step" -> [w57] mode=indexing
        shift-right: [w61] -> _
        shift-left: cluster{dbl, "Field Reading":dbl}[] [] -> [w62]
        shift-right: [w56] -> _
        shift-left: w50 -> [w63]
        shift-right: [w54] -> _
        shift-left: cluster{dbl, "Field Reading":dbl}[] [] -> [w55]
        n23 = call "Build_serie_EL.vi"("end value"=w58, "increment"=w57, "start value"=w59) -> ("output array"=w60:dbl[])
        n24 = for {
          tunnel: w60 -> [w69] mode=indexing
          shift-right: [w67] -> w61
          shift-left: w62 -> [w68]
          shift-right: [w66] -> w56
          shift-left: w63 -> [w70]
          shift-right: [w64] -> w54
          shift-left: w55 -> [w65]
          n25 = stacked-sequence {
            tunnel: w70 -> [w71 _ w82 _]
            tunnel: w68 -> [_ _ w87 _]
            tunnel: w69 -> [w72 _ _ _]
            tunnel: [_ _ w86 _] -> w67
            tunnel: [_ _ w81 _] -> w66
            tunnel: w65 -> [_ _ w78 _]
            tunnel: [_ _ w77 _] -> w64
            frame #0 {
              n26 = call <instrlib>:"Configure Source (Level).vi"("VISA resource name"=w71, "Source Measure Unit Channel (0: Channel A)"=0, "Level Type (1: Voltage)"=1, "Voltage Level (0 V)"=w72) -> ()  [unwired: 10 in, 2 out]
            }
            frame #1 {
              n27 = Wait (ms)(milliseconds to wait="Wait (ms)") -> ()  [unwired: 1 out]
            }
            frame #2 {
              n28 = call-poly <instrlib>:"Read Measurement.vi"("Wait Time (10 S)"=0, "Source Measure Unit Channel (0: Channel A)"=0, "VISA resource name"=w82) -> ("Last Voltage (V)"=w79:dbl, "Last Current (A)"=w83:dbl, "VISA resource name out"=w81:refnum<visa-resource-name>)  [unwired: 3 in, 3 out]
              "Current (A)" <- w83
              "Voltage (V)" <- w79
              n29 = Bundle("Last Voltage (V)"=w79, "Last Current (A)"=w83) -> (w88:T2)  [unwired: 1 in]
              n30 = Divide(x=w79, y=w83) -> (x/y=w76:dbl)
              "Resistance (ohm)" <- w76
              n31 = Build Array(w79, w83, w76) -> (→"data":dbl[])
              n32 = Build Array (concatenate)(w87, w88) -> (w86:T3)
              "I vs V" <- w86
              n33 = Bundle("Last Voltage (V)"=w79, w76) -> (w80:cluster{"Last Voltage (V)":dbl, dbl})  [unwired: 1 in]
              n34 = Build Array (concatenate)(w78, w80) -> (w77:T4)
              "R vs V" <- w77
            }
            frame #3 {
              n35 = local read "data"() -> (w90:dbl[])
              n36 = Array To Spreadsheet String(array=w90, 3:"%e" ("format string")) -> (spreadsheet string=w93:string)  [unwired: 1 in]
              n37 = local read "File path"() -> (w92:path)
              n38 = call <vilib>:"Write Characters To File.vi"("append to file? (new file:F)"=TRUE, "character string"=w93, "file path (dialog if empty)"=w92) -> ()  [unwired: 2 in, 1 out]
            }
          }
        }
      }
    }
    frame #4 {
      w97 = 0
      n39 = call <instrlib>:"Configure Source (Level).vi"("VISA resource name"=w98, "Source Measure Unit Channel (0: Channel A)"=w97, "Level Type (1: Voltage)"=1, "Voltage Level (0 V)"=0.0) -> ("VISA resource name out"=w100:refnum<visa-resource-name>)  [unwired: 10 in, 1 out]
      n40 = call <instrlib>:"Enable Source Output.vi"("Output Mode (0: Turn off)"=w97, "Source Measure Unit Channel (0: Channel A)"=w97, "VISA resource name"=w100) -> ("VISA resource name out"=w95:refnum<visa-resource-name>)  [unwired: 7 in, 1 out]
      n41 = call <instrlib>:"Close.vi"("VISA resource name"=w95) -> ()  [unwired: 10 in, 1 out]
    }
  }
